vi "VP_NanoPositioner_FPGA.vi"() -> ()   [LabVIEW 2015]
uses:
  FPGA states.ctl
  FPGA Commands.ctl
  <vilib>/Platform/TimedLoop/XDataNode/timing_clust.ctl
  <vilib>/Platform/TimedLoop/XDataNode/nitl_modes.ctl
  <vilib>/Platform/TimedLoop/XDataNode/wakeup.ctl
  Control X Up Down Ramp.ctl
  Control Y Up Down Ramp.ctl
  Detector_Trigger_Control.ctl
  <vilib>/rvi/Emulation/niFpgaGetClockAttributes.vi
  <vilib>/rvi/Emulation/niFpgaSctlEmulationGetInTimedLoop.vi
  <vilib>/rvi/Emulation/niFpgaEmulationReportErrorSimple.vi
  <vilib>/rvi/eio/common/nirviEmuTemplateMethod_errors.vi
  <vilib>/rvi/Emulation/niFpgaProcessEmulError.vi
  <vilib>/rvi/Emulation/niFpgaCriticalErrorInLSC.vi
  <vilib>/rvi/interface/RandomDataEmulation/niFpgaRandomDataHandleErrors.vi
  <vilib>/eio/EIONode/EIONode.xnode
  <vilib>/rvi/DataTransferAndStorage/Container/XNode/niFpgaContainer.xnode
  <vilib>/rvi/interface/RandomDataEmulation/nirviRandomDataFpgaReadWriteTemplate.vi
  <vilib>/rvi/Analysis/measure/butterworth/XNode/niFpgaButterworthFilter.xnode
  <vilib>/Platform/TimedLoop/XDataNode/XDataNode.xnode
  <vilib>/Platform/TimedLoop/XDataNode/XDNodeRunTimeDep.lvlib
panel:
  out "Fly scan completed":bool
  out "Y scan done":bool=TRUE
  out "X scan done":bool=TRUE
  out "Wait error":errorcluster
  out "Shutdown error":errorcluster
  out "FPGA error monitor":errorcluster
  out "Run Loop error":errorcluster
  in  "Wait timer (ms)":u16=50 caption="Count(mSec)"
  in  "New FPGA command":bool
  in  "FPGA command":T1
  out "FPGA state":T2
  out "End Run Error":errorcluster
  out "Number of Data Strings 2":i32
  out "Measured Data Trigger Time Period (Ticks)":u32
  in  "Data Trigger Time Period (uSec)":u32 caption="Detector Trigger Time Period (uSec)"
  out "Trigger for Data":fxp<+/-,58,25>
  out "Fly Scan Running":bool
  in  "Fly Scan":bool
  out "If True End Y Down Ramp":bool
  in  "Y Ramp Drop Size (nm)":fxp<+/-,16,16>
  out "Ramp Mid Range":bool
  out "If True End Up Ramp":bool
  out "Start or middle":bool=TRUE
  in  "Y Start Marker (nm)":fxp<+/-,58,25> format="%#_55g"
  out "Y Ramp Slope":fxp<+,48,16>
  in  "Y Ramp End (nm)":fxp<+/-,16,16>
  in  "Y Ramp Start (nm)":fxp<+/-,16,16>
  in  "Y Ramp Period (usec)":fxp<+,32,32>
  in  "X Ramp Period (usec)":fxp<+,32,32>
  in  "X Ramp End (nm)":fxp<+/-,16,16>
  in  "X Ramp Start (nm)":fxp<+/-,16,16>
  out "If True End X Down Ramp":bool
  out "X Ramp Mid Range":bool
  out "If True End X Up Ramp":bool
  out "Y Ramp Drop":bool
  out "Next Do Down Ramp":bool
  out "Continue Run":bool
  in  "X Start Marker (nm)":fxp<+/-,58,25>
  out "X Ramp Slope":fxp<+,48,16> format="%.37g"
  in  "DT Reset":bool
  in  "DT Duty Cycle (periods)":fxp<+,32,0>=0.5 caption="DT duty cycle (periods)"
  in  "DT Reference DC Offset (V)":fxp<+/-,16,16>
  in  "DT Reference Amplitude (V)":fxp<+/-,40,17>
  in  "DT Phase Offset (periods)":fxp<+,32,0>
  in  "DT Frequency (periods/tick)":fxp<+,32,0>=0.0002500000409781933
  in  "Trigger Wave Generator":T3(ring)
  out "If True End Trigger Low":bool
  in  "Trigger Low Level (V)":fxp<+/-,20,5>=-5.0
  in  "Trigger High Level (V)":fxp<+/-,20,5>=5.0
  out "If True End Trigger High":bool
  out "Trigger Mid High":bool
  in  "Trigger Low Period (usec)":fxp<+/-,64,45>
  in  "Trigger High Period (usec)":fxp<+/-,64,45>
  out "Measured Z Reference Time Period (Ticks)":u32
  in  "Z Reference Time Period (uSec)":u32
  in  "Z White Noise Amplitude":u16=32767
  in  "Z White Noise Seed":u32=4
  in  "Z Phase Offset (periods)":fxp<+,32,0>
  in  "Z Frequency (periods/tick)":fxp<+,32,0>=0.0002500000409781933
  in  "Z Reference DC Offset (nm)":fxp<+/-,16,16>
  in  "Z Reference Amplitude (nm)":fxp<+/-,40,17>
  in  "Z Reference Reset":bool
  in  "Z Reference Wave Selection":T4(ring)
  in  "Y White Noise Amplitude":u16=32767
  in  "Y White Noise Seed":u32=4
  out "Measured Y Reference Time Period (Ticks)":u32
  in  "Y Reference Time Period (uSec)":u32
  in  "Y Reference Reset":bool
  in  "Y Reference Wave Selection":T5(ring)
  in  "Detector Trigger Lower Limit (V)":fxp<+/-,20,5>=-5.0
  out "Detector Trigger In Range?":bool
  in  "Detector Trigger Upper Limit (V)":fxp<+/-,20,5>=5.0
  out "Detector Trigger (V)":fxp<+/-,20,5> format="%.29g"
  out "Measured Detector Trigger Time Period (Ticks)":u32
  in  "Detector Trigger Time Period (uSec)":u32
  out "Measured Trigger Gen Time Period (Ticks)":u32
  in  "Trigger Generation Time Period (uSec)":u32
  in  "Reference Signal Source":T6(ring)
  in  "Z-Stage Scaling Direction":fxp<+/-,3,3>=-1.0
  in  "Y-Stage Scaling Direction":fxp<+/-,3,3>=-1.0
  in  "Y Phase Offset (periods)":fxp<+,32,0>
  in  "Y Frequency (periods/tick)":fxp<+,32,0>=0.0002500000409781933
  in  "Optics and or Sample Stage":T7(ring)
  out "Z Stage External Reference (nm)":fxp<+/-,58,25>
  in  "Mod 3 AI2 V to nm Scaling":fxp<+,47,18>
  out "Mod 8 Input AI2 (V)":fxp<+/-,24,5>
  out "Y Stage External Reference (nm)":fxp<+/-,58,25>
  in  "Mod 3 AI1 V to nm Scaling":fxp<+,47,18>
  out "Mod 8 Input AI1 (V)":fxp<+/-,24,5>
  in  "Sample Z Stage Resolution (nm)":fxp<+,33,3>=0.001000046730041504
  in  "Sample Y Stage Resolution (nm)":fxp<+,33,3>=0.001000046730041504
  in  "Sample X Stage Resolution (nm)":fxp<+,33,3>=0.001000046730041504
  out "Sample Z Stage Displacement (nm)":fxp<+/-,58,25>
  out "Sample Z Stage Displacement raw (nm)":fxp<+/-,64,35> format="%.62g"
  out "Sample Y Stage Displacement (nm)":fxp<+/-,58,25>
  out "Sample Y Stage Displacement raw (nm)":fxp<+/-,64,35> format="%.41g"
  out "Sample X Stage Displacement raw (nm)":fxp<+/-,64,35> format="%.62g"
  out "Sample X Stage Displacement (nm)":fxp<+/-,58,25>
  in  "Reset Sample Z":bool
  out "32 bit Count Sample  Z":i32
  in  "Reset Sample Y":bool
  out "32 bit Count Sample  Y":i32
  in  "Reset Sample X":bool
  out "32 bit Count Sample X":i32
  out "Mod6/DIO3":bool
  out "Mod6/DIO2":bool
  out "Mod5/DIO3":bool
  out "Mod5/DIO2":bool
  out "Mod4/DIO3":bool
  out "Mod4/DIO2":bool
  out "Measured Analog Input Time Period (Ticks)":u32
  in  "Analog Input Time Period (uSec)":u32
  out "X Stage External Reference (nm)":fxp<+/-,58,25>
  in  "Mod 3 AI0 V to nm Scaling":fxp<+,47,18>
  out "Mod 3 Input AI0 (V)":fxp<+/-,24,5>
  out "Kxz Output, Kxz*ex (V)":fxp<+/-,58,25> format="%.31g"
  out "Kyz Output, Kyz*ey (V)":fxp<+/-,58,25> format="%.31g"
  in  "b02(2) yz1":fxp<+/-,64,9>[](array[numeric])=[0.0, 0.0, 0.0, 0.0, 0.0, 0.0, 0.0, 0.0, 0.0, 0.0, 0.0, 0.0, 0.0, 0.0, 0.0, 0.0, 0.0, 0.0, 0.0, 0.0]
  in  "b01(2) yz1":fxp<+/-,64,9>[](array[numeric])=[0.0, 0.0, 0.0, 0.0, 0.0, 0.0, 0.0, 0.0, 0.0, 0.0, 0.0, 0.0, 0.0, 0.0, 0.0, 0.0, 0.0, 0.0, 0.0, 0.0]
  in  "-a02(2) yz1":fxp<+/-,64,9>[](array[numeric])=[0.0, 0.0, 0.0, 0.0, 0.0, 0.0, 0.0, 0.0, 0.0, 0.0, 0.0, 0.0, 0.0, 0.0, 0.0, 0.0, 0.0, 0.0, 0.0, 0.0]
  in  "-a01(2) yz1":fxp<+/-,64,9>[](array[numeric])=[0.0, 0.0, 0.0, 0.0, 0.0, 0.0, 0.0, 0.0, 0.0, 0.0, 0.0, 0.0, 0.0, 0.0, 0.0, 0.0, 0.0, 0.0, 0.0, 0.0]
  in  "sos gain SF Controller yz1":fxp<+/-,42,9>
  in  "b02(2) xz1":fxp<+/-,64,9>[](array[numeric])=[0.0, 0.0, 0.0, 0.0, 0.0, 0.0, 0.0, 0.0, 0.0, 0.0, 0.0, 0.0, 0.0, 0.0, 0.0, 0.0, 0.0, 0.0, 0.0, 0.0]
  in  "b01(2) xz1":fxp<+/-,64,9>[](array[numeric])=[0.0, 0.0, 0.0, 0.0, 0.0, 0.0, 0.0, 0.0, 0.0, 0.0, 0.0, 0.0, 0.0, 0.0, 0.0, 0.0, 0.0, 0.0, 0.0, 0.0]
  in  "-a02(2) xz1":fxp<+/-,64,9>[](array[numeric])=[0.0, 0.0, 0.0, 0.0, 0.0, 0.0, 0.0, 0.0, 0.0, 0.0, 0.0, 0.0, 0.0, 0.0, 0.0, 0.0, 0.0, 0.0, 0.0, 0.0]
  in  "-a01(2) xz1":fxp<+/-,64,9>[](array[numeric])=[0.0, 0.0, 0.0, 0.0, 0.0, 0.0, 0.0, 0.0, 0.0, 0.0, 0.0, 0.0, 0.0, 0.0, 0.0, 0.0, 0.0, 0.0, 0.0, 0.0]
  in  "sos gain SF Controller xz1":fxp<+/-,42,9>
  out "Kzy Output, Kzy*ez (V)":fxp<+/-,58,25> format="%.31g"
  out "Kxy Output, Kxy*ex (V)":fxp<+/-,58,25> format="%.31g"
  in  "b02(2) zy1":fxp<+/-,64,9>[](array[numeric])=[0.0, 0.0, 0.0, 0.0, 0.0, 0.0, 0.0, 0.0, 0.0, 0.0, 0.0, 0.0, 0.0, 0.0, 0.0, 0.0, 0.0, 0.0, 0.0, 0.0]
  in  "b01(2) zy1":fxp<+/-,64,9>[](array[numeric])=[0.0, 0.0, 0.0, 0.0, 0.0, 0.0, 0.0, 0.0, 0.0, 0.0, 0.0, 0.0, 0.0, 0.0, 0.0, 0.0, 0.0, 0.0, 0.0, 0.0]
  in  "-a02(2) zy1":fxp<+/-,64,9>[](array[numeric])=[0.0, 0.0, 0.0, 0.0, 0.0, 0.0, 0.0, 0.0, 0.0, 0.0, 0.0, 0.0, 0.0, 0.0, 0.0, 0.0, 0.0, 0.0, 0.0, 0.0]
  in  "-a01(2) zy1":fxp<+/-,64,9>[](array[numeric])=[0.0, 0.0, 0.0, 0.0, 0.0, 0.0, 0.0, 0.0, 0.0, 0.0, 0.0, 0.0, 0.0, 0.0, 0.0, 0.0, 0.0, 0.0, 0.0, 0.0]
  in  "sos gain SF Controller zy1":fxp<+/-,42,9>
  in  "b02(2) xy1":fxp<+/-,64,9>[](array[numeric])=[0.0, 0.0, 0.0, 0.0, 0.0, 0.0, 0.0, 0.0, 0.0, 0.0, 0.0, 0.0, 0.0, 0.0, 0.0, 0.0, 0.0, 0.0, 0.0, 0.0]
  in  "b01(2) xy1":fxp<+/-,64,9>[](array[numeric])=[0.0, 0.0, 0.0, 0.0, 0.0, 0.0, 0.0, 0.0, 0.0, 0.0, 0.0, 0.0, 0.0, 0.0, 0.0, 0.0, 0.0, 0.0, 0.0, 0.0]
  in  "-a02(2) xy1":fxp<+/-,64,9>[](array[numeric])=[0.0, 0.0, 0.0, 0.0, 0.0, 0.0, 0.0, 0.0, 0.0, 0.0, 0.0, 0.0, 0.0, 0.0, 0.0, 0.0, 0.0, 0.0, 0.0, 0.0]
  in  "-a01(2) xy1":fxp<+/-,64,9>[](array[numeric])=[0.0, 0.0, 0.0, 0.0, 0.0, 0.0, 0.0, 0.0, 0.0, 0.0, 0.0, 0.0, 0.0, 0.0, 0.0, 0.0, 0.0, 0.0, 0.0, 0.0]
  in  "sos gain SF Controller xy1":fxp<+/-,42,9>
  out "Kzx Output, Kzx*ez (V)":fxp<+/-,58,25> format="%.31g"
  in  "b02(2) zx1":fxp<+/-,64,9>[](array[numeric])=[0.0, 0.0, 0.0, 0.0, 0.0, 0.0, 0.0, 0.0, 0.0, 0.0, 0.0, 0.0, 0.0, 0.0, 0.0, 0.0, 0.0, 0.0, 0.0, 0.0]
  in  "b01(2) zx1":fxp<+/-,64,9>[](array[numeric])=[0.0, 0.0, 0.0, 0.0, 0.0, 0.0, 0.0, 0.0, 0.0, 0.0, 0.0, 0.0, 0.0, 0.0, 0.0, 0.0, 0.0, 0.0, 0.0, 0.0]
  in  "-a02(2) zx1":fxp<+/-,64,9>[](array[numeric])=[0.0, 0.0, 0.0, 0.0, 0.0, 0.0, 0.0, 0.0, 0.0, 0.0, 0.0, 0.0, 0.0, 0.0, 0.0, 0.0, 0.0, 0.0, 0.0, 0.0]
  in  "-a01(2) zx1":fxp<+/-,64,9>[](array[numeric])=[0.0, 0.0, 0.0, 0.0, 0.0, 0.0, 0.0, 0.0, 0.0, 0.0, 0.0, 0.0, 0.0, 0.0, 0.0, 0.0, 0.0, 0.0, 0.0, 0.0]
  in  "sos gain SF Controller zx1":fxp<+/-,42,9>
  out "Kyx Output, Kyx*ey (V)":fxp<+/-,58,25> format="%.31g"
  in  "b02(2) yx1":fxp<+/-,64,9>[](array[numeric])=[0.0, 0.0, 0.0, 0.0, 0.0, 0.0, 0.0, 0.0, 0.0, 0.0, 0.0, 0.0, 0.0, 0.0, 0.0, 0.0, 0.0, 0.0, 0.0, 0.0]
  in  "b01(2) yx1":fxp<+/-,64,9>[](array[numeric])=[0.0, 0.0, 0.0, 0.0, 0.0, 0.0, 0.0, 0.0, 0.0, 0.0, 0.0, 0.0, 0.0, 0.0, 0.0, 0.0, 0.0, 0.0, 0.0, 0.0]
  in  "-a02(2) yx1":fxp<+/-,64,9>[](array[numeric])=[0.0, 0.0, 0.0, 0.0, 0.0, 0.0, 0.0, 0.0, 0.0, 0.0, 0.0, 0.0, 0.0, 0.0, 0.0, 0.0, 0.0, 0.0, 0.0, 0.0]
  in  "-a01(2) yx1":fxp<+/-,64,9>[](array[numeric])=[0.0, 0.0, 0.0, 0.0, 0.0, 0.0, 0.0, 0.0, 0.0, 0.0, 0.0, 0.0, 0.0, 0.0, 0.0, 0.0, 0.0, 0.0, 0.0, 0.0]
  in  "sos gain SF Controller yx1":fxp<+/-,42,9>
  in  "X-Stage Scaling Direction":fxp<+/-,3,3>=-1.0
  in  "Z-Stage nm to V Scaling":fxp<+/-,32,12>
  in  "Y-Stage nm to V Scaling":fxp<+/-,32,12>
  in  "X-Stage nm to V Scaling":fxp<+/-,32,12>
  out "Kxx Output, Kxx*ex (V)":fxp<+/-,58,25>
  out "Kyy Output, Kyy*ey (V)":fxp<+/-,58,25>
  out "Kzz Output, Kzz*ez (V)":fxp<+/-,58,25>
  in  "sos gain SF Controller xx1":fxp<+/-,42,9>
  in  "-a01(2) xx1":fxp<+/-,64,9>[](array[numeric])=[0.0, 0.0, 0.0, 0.0, 0.0, 0.0, 0.0, 0.0, 0.0, 0.0, 0.0, 0.0, 0.0, 0.0, 0.0, 0.0, 0.0, 0.0, 0.0, 0.0]
  in  "-a02(2) xx1":fxp<+/-,64,9>[](array[numeric])=[0.0, 0.0, 0.0, 0.0, 0.0, 0.0, 0.0, 0.0, 0.0, 0.0, 0.0, 0.0, 0.0, 0.0, 0.0, 0.0, 0.0, 0.0, 0.0, 0.0]
  in  "b01(2) xx1":fxp<+/-,64,9>[](array[numeric])=[0.0, 0.0, 0.0, 0.0, 0.0, 0.0, 0.0, 0.0, 0.0, 0.0, 0.0, 0.0, 0.0, 0.0, 0.0, 0.0, 0.0, 0.0, 0.0, 0.0]
  in  "b02(2) xx1":fxp<+/-,64,9>[](array[numeric])=[0.0, 0.0, 0.0, 0.0, 0.0, 0.0, 0.0, 0.0, 0.0, 0.0, 0.0, 0.0, 0.0, 0.0, 0.0, 0.0, 0.0, 0.0, 0.0, 0.0]
  in  "sos gain SF Controller yy1":fxp<+/-,42,9>
  in  "-a01(2) yy1":fxp<+/-,64,9>[](array[numeric])=[0.0, 0.0, 0.0, 0.0, 0.0, 0.0, 0.0, 0.0, 0.0, 0.0, 0.0, 0.0, 0.0, 0.0, 0.0, 0.0, 0.0, 0.0, 0.0, 0.0]
  in  "-a02(2) yy1":fxp<+/-,64,9>[](array[numeric])=[0.0, 0.0, 0.0, 0.0, 0.0, 0.0, 0.0, 0.0, 0.0, 0.0, 0.0, 0.0, 0.0, 0.0, 0.0, 0.0, 0.0, 0.0, 0.0, 0.0]
  in  "b01(2) yy1":fxp<+/-,64,9>[](array[numeric])=[0.0, 0.0, 0.0, 0.0, 0.0, 0.0, 0.0, 0.0, 0.0, 0.0, 0.0, 0.0, 0.0, 0.0, 0.0, 0.0, 0.0, 0.0, 0.0, 0.0]
  in  "b02(2) yy1":fxp<+/-,64,9>[](array[numeric])=[0.0, 0.0, 0.0, 0.0, 0.0, 0.0, 0.0, 0.0, 0.0, 0.0, 0.0, 0.0, 0.0, 0.0, 0.0, 0.0, 0.0, 0.0, 0.0, 0.0]
  in  "sos gain SF Controller zz1":fxp<+/-,42,9>
  in  "-a01(2) zz1":fxp<+/-,64,9>[](array[numeric])=[0.0, 0.0, 0.0, 0.0, 0.0, 0.0, 0.0, 0.0, 0.0, 0.0, 0.0, 0.0, 0.0, 0.0, 0.0, 0.0, 0.0, 0.0, 0.0, 0.0]
  in  "-a02(2) zz1":fxp<+/-,64,9>[](array[numeric])=[0.0, 0.0, 0.0, 0.0, 0.0, 0.0, 0.0, 0.0, 0.0, 0.0, 0.0, 0.0, 0.0, 0.0, 0.0, 0.0, 0.0, 0.0, 0.0, 0.0]
  in  "b01(2) zz1":fxp<+/-,64,9>[](array[numeric])=[0.0, 0.0, 0.0, 0.0, 0.0, 0.0, 0.0, 0.0, 0.0, 0.0, 0.0, 0.0, 0.0, 0.0, 0.0, 0.0, 0.0, 0.0, 0.0, 0.0]
  in  "b02(2) zz1":fxp<+/-,64,9>[](array[numeric])=[0.0, 0.0, 0.0, 0.0, 0.0, 0.0, 0.0, 0.0, 0.0, 0.0, 0.0, 0.0, 0.0, 0.0, 0.0, 0.0, 0.0, 0.0, 0.0, 0.0]
  in  "Scaling mV to V":fxp<+,33,10>=0.0009765625
  in  "System Loop Type":enum16{"Open Loop", "Closed Loop"}(ring)
  in  "Timeout FPGA FIFO1":i32=40000000
  out "FIFO Timed Out":bool
  out "Number of Data Strings":i32
  in  "Y Reference DC Offset (nm)":fxp<+/-,16,16>
  in  "X Reference DC Offset (nm)":fxp<+/-,16,16>
  in  "Y Reference Amplitude (nm)":fxp<+/-,40,17>
  out "Z Stage Reference (nm)":fxp<+/-,58,25> format="%.41g"
  out "Y Stage Reference (nm)":fxp<+/-,58,25> format="%.41g"
  out "Optics Z Stage Displacement (nm)":fxp<+/-,58,25>
  out "Optics Z Stage Displacement raw (nm)":fxp<+/-,64,35>
  in  "Optics Z Stage Resolution (nm)":fxp<+,33,3>=0.001000046730041504
  in  "Reset Optics Z":bool
  out "32 bit Count Optics  Z":i32
  out "Mod6/DIO1":bool
  out "Mod6/DIO0":bool
  out "Optics Y Stage Displacement (nm)":fxp<+/-,58,25>
  out "Optics Y Stage Displacement raw (nm)":fxp<+/-,64,35>
  in  "Optics Y Stage Resolution (nm)":fxp<+,33,3>=0.001000046730041504
  in  "Reset Optics Y":bool
  out "32 bit Count Optics  Y":i32
  out "Mod5/DIO1":bool
  out "Mod5/DIO0":bool
  out "Z-Stage Input In Range?":bool
  out "Y-Stage Input In Range?":bool
  in  "Controller Output Lower Limit":fxp<+/-,20,5>=-5.0
  out "X-Stage Input In Range?":bool
  in  "Controller Output Upper Limit":fxp<+/-,20,5>=5.0
  in  "X White Noise Amplitude":u16=32767
  in  "X White Noise Seed":u32=4
  in  "X Reference Reset":bool
  in  "X Reference Wave Selection":T8(ring)
  out "Measured Counter Time Period (Ticks)":u32
  out "Measured Datalog Time Period (Ticks)":u32
  out "Measured Plant Output Time Period (Ticks)":u32
  out "Measured Controller Output Time Period (Ticks)":u32
  out "Measured Controller Time Period (Ticks)":u32
  out "Measured X Reference Time Period (Ticks)":u32
  out "Optics X Stage Displacement raw (nm)":fxp<+/-,64,35>
  in  "Optics X Stage Resolution (nm)":fxp<+,33,3>=0.001000046730041504 format="%#_31g"
  in  "Plant Output Time Period (uSec)":u32
  out "Optics X Stage Displacement (nm)":fxp<+/-,58,25>
  in  "Reset Optics X":bool
  out "32 bit Count Optics X":i32
  out "Mod4/DIO1":bool
  out "Mod4/DIO0":bool
  out "Start Run Error":errorcluster
  out "stop case":bool
  in  "Controller Output Time Period (uSec)":u32
  in  "Datalog Cases":T9(ring)
  out "PI Z-Stage Input (V)":fxp<+/-,20,5> format="%.29g"
  out "PI Y-Stage Input (V)":fxp<+/-,20,5> format="%.29g"
  out "PI X-Stage Input (V)":fxp<+/-,20,5> format="%.29g"
  in  "Controller Time Period (uSec)":u32
  in  "Datalog Time Period (uSec)":u32
  in  "X Reference Time Period (uSec)":u32
  in  "X Reference Amplitude (nm)":fxp<+/-,40,17>
  out "X Stage Reference (nm)":fxp<+/-,58,25> format="%.41g"
  out "FIFO Timed Out?":bool
  in  "X Phase Offset (periods)":fxp<+,32,0>
  in  "X Frequency (periods/tick)":fxp<+,32,0>=0.0002500000409781933
types:
  T1 = typedef "FPGA Commands.ctl" = enum16{"Start Scan", "Shutdown"}
  T2 = typedef "FPGA states.ctl" = enum16{"Wait", "Start Run", "Run", "End Run", "Shutdown"}
  T3 = enum16{"Custom Square Wave ", "Square Wave 1", "Square Wave 2"}
  T4 = enum16{"Constant", "Sine Wave", "Sawtooth Wave", "Square Wave", "Filtered White Noise"}
  T5 = enum16{"Constant", "Sine Wave", "Custom Ramp Wave", "Filtered White Noise"}
  T6 = enum16{"FPGA Generated Reference", "External Reference"}
  T7 = enum16{"Optics Stage Only", "Optics and Sample Stage"}
  T8 = enum16{"Constant", "Sine Wave", "Custom Up Down Ramp", "Filtered White Noise"}
  T9 = enum16{"Data Log 1", "Data Log 2", "Data Log 3", "Data Log 4", "Data Log 5", "Data Log 6", "Data Log 7", "Data Log 8", "Data Log 9", "Data Log 10", "Data Log 11", "Data Log 12", "Data Log 13", "Data Log 14", "Data Log 15", "Data Log 16"}
  T10 = typedef "Control Y Up Down Ramp.ctl" = enum16{"Y Up Ramp", "Y Down Ramp"}
  T11 = typedef "Detector_Trigger_Control.ctl" = enum16{"Trigger High", "Trigger Low"}
  T12 = typedef "XDNodeRunTimeDep.lvlib/timing_clust.ctl" = cluster{"Expected End [f-1]":u64, "Actual End [f-1]":u64, "Finished Late? [f-1]":bool, "Expected End [i-1]":u64, "Actual End [i-1]":u64, "Finished Late? [i-1]":bool, "Expected Start [i]":u64, "Actual Start [i]":u64, "Expected Start [f]":u64, "Actual Start [f]":u64, "Source Name":string, "Structure Name":string, "Period":i64, "Deadline":i64, "Offset":i64, "Start":i64, "Priority":i32, "Timeout":i32, "Mode":T13, "Wakeup Reason":T14, "Error":errorcluster, "Source Type":string, "Secondary Source Type":string, "Global End Time":u64, "Global Start Time":u64, "Frame Duration":u64, "Iteration Duration":u64, "Assigned CPU":i32, "I/O Scan Engine Mode":u32}
  T13 = typedef "XDNodeRunTimeDep.lvlib/nitl_modes.ctl" = enum32{"No Change", "Process missed periods, maintain original phase", "Discard missed periods, maintain original phase", "Process missed periods, ignore original phase", "Discard missed periods, ignore original phase"}
  T14 = typedef "XDNodeRunTimeDep.lvlib/wakeup.ctl" = enum32{"Normal", "Aborted", "Asynchronous wakeup", "Timing source error", "Timed loop error", "Timeout"}
  T15 = typedef "Control X Up Down Ramp.ctl" = enum16{"X Up Ramp", "X Down Ramp"}
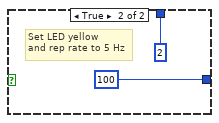
[diagram p2: hidden frame]
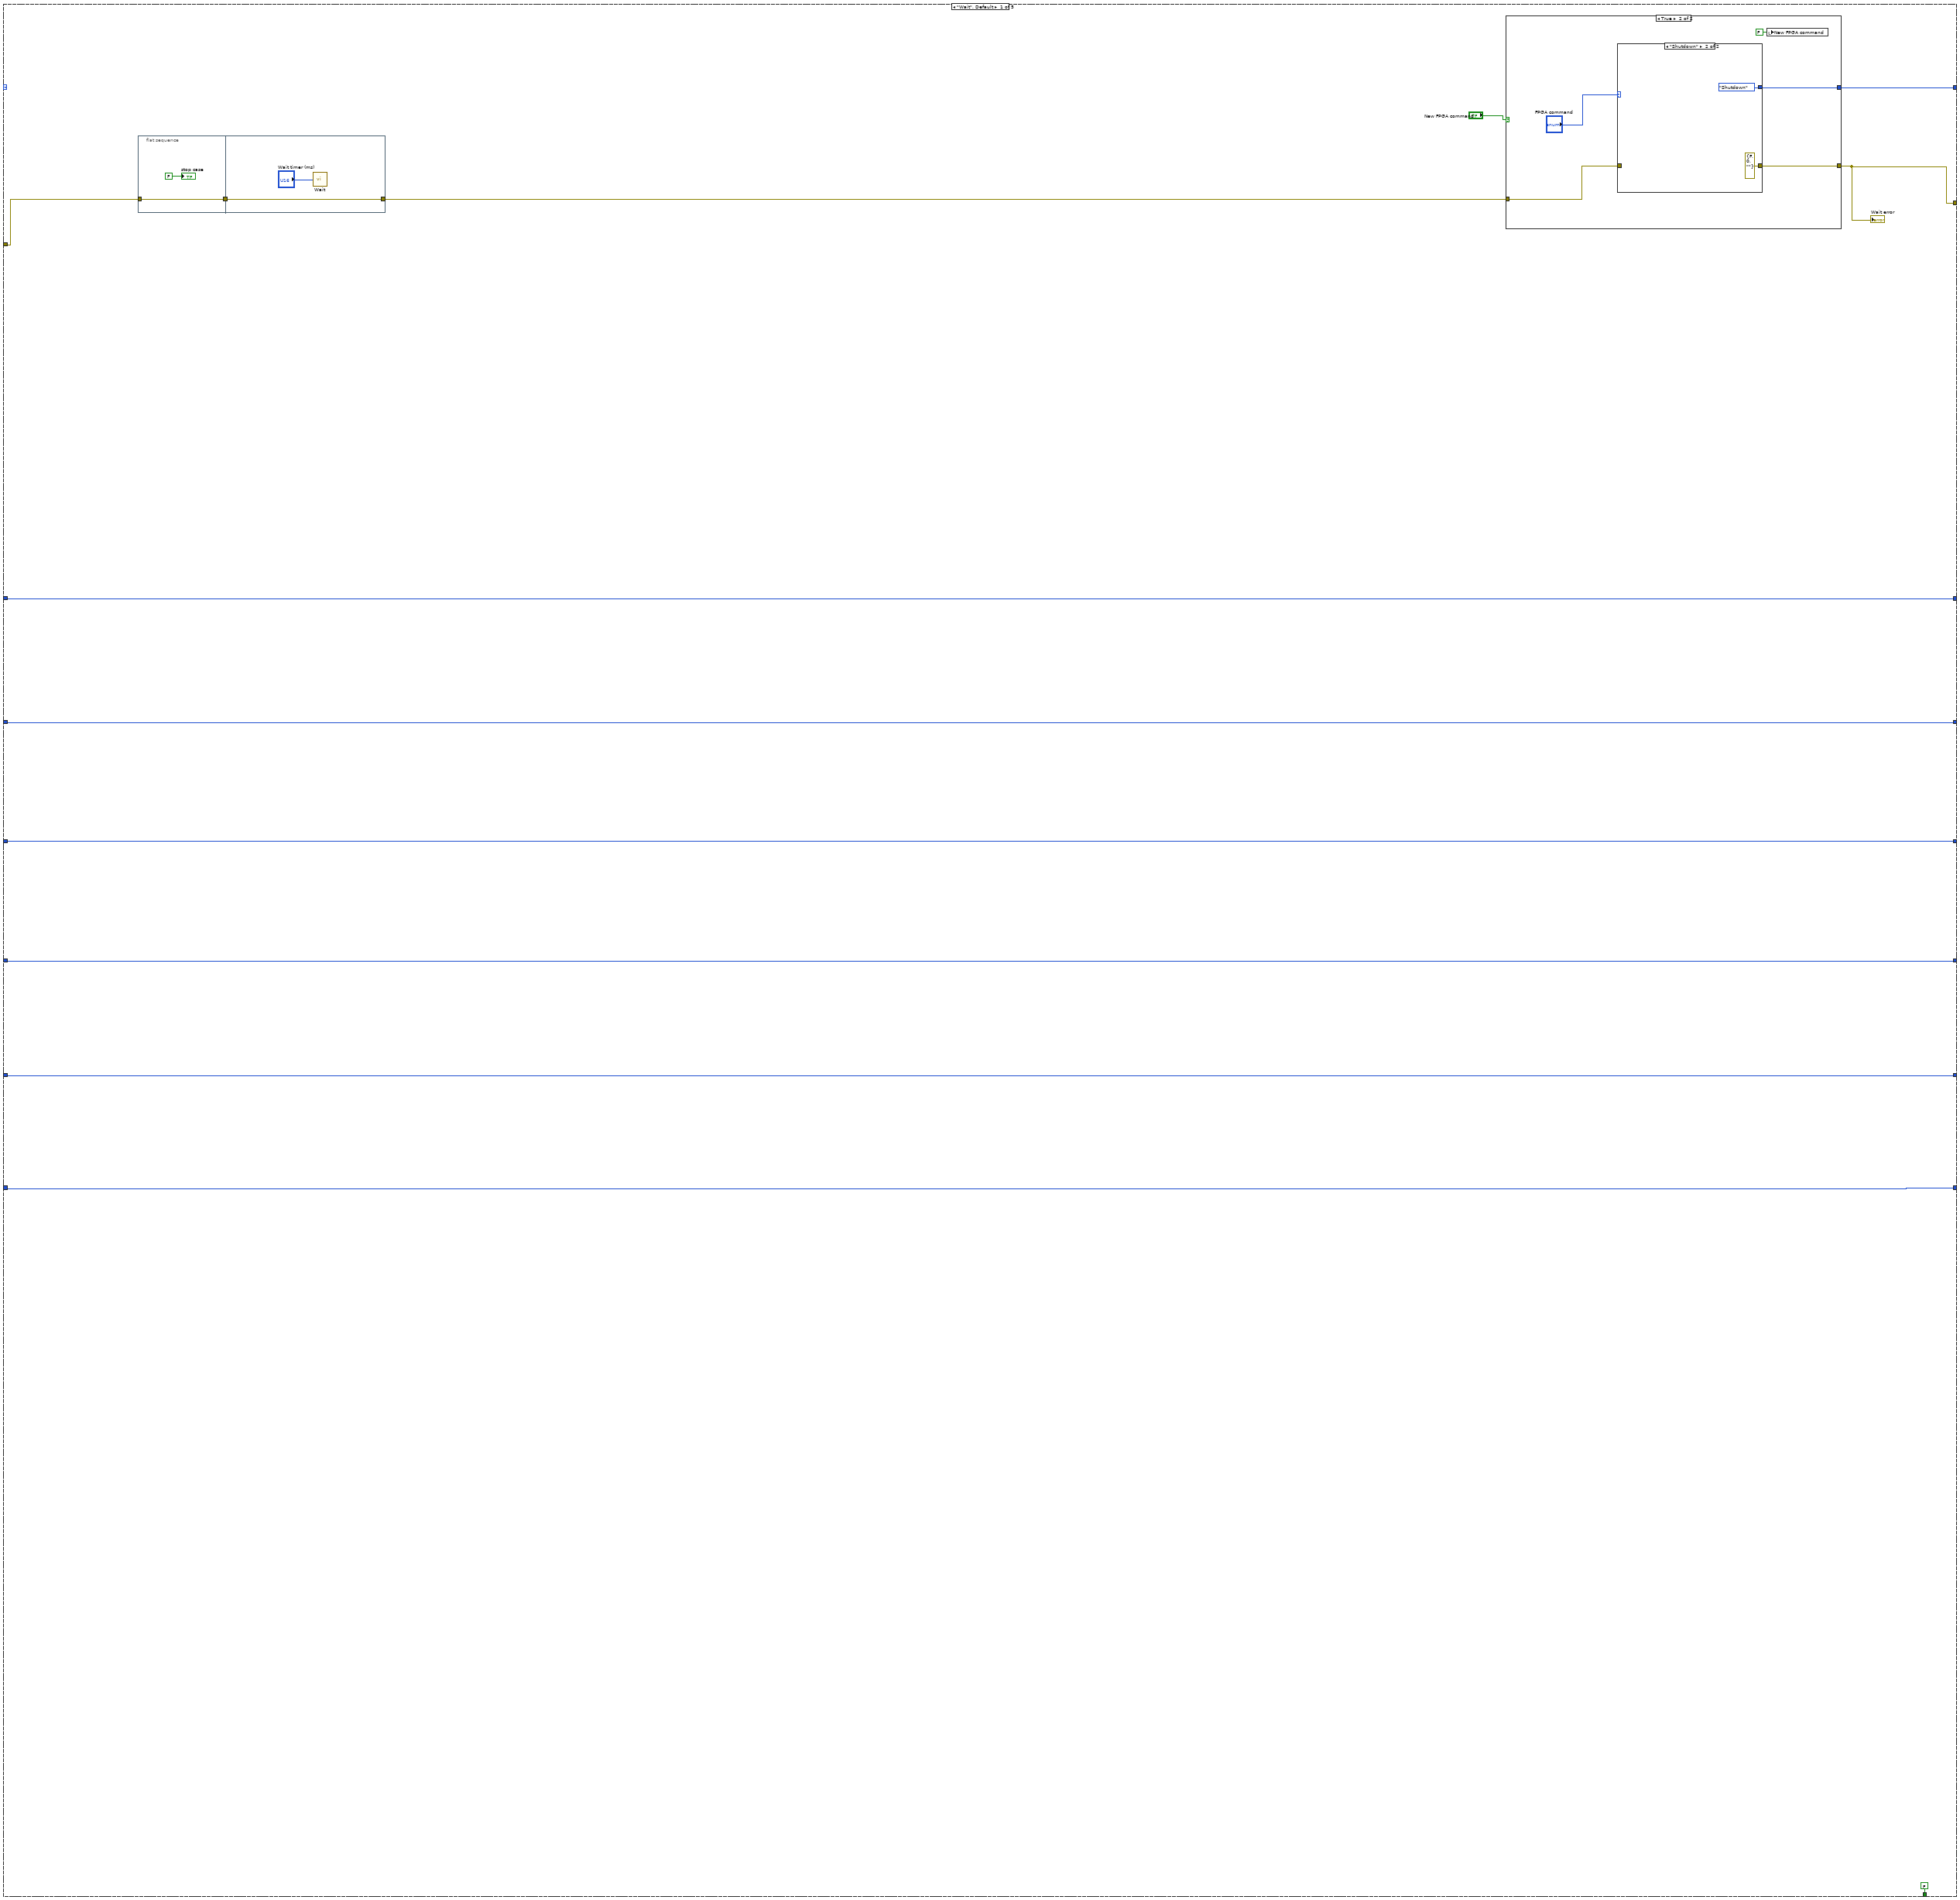
[diagram p3: hidden frame]
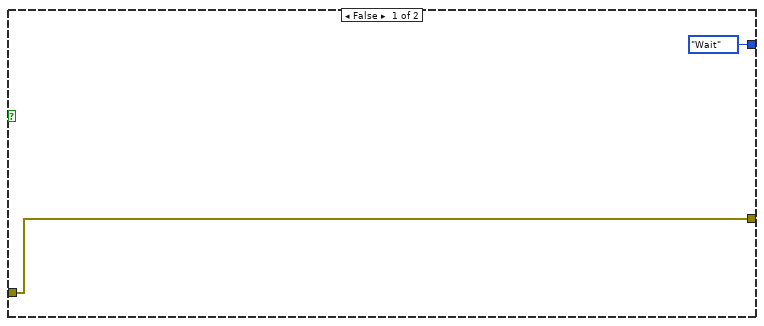
[diagram p4: hidden frame]
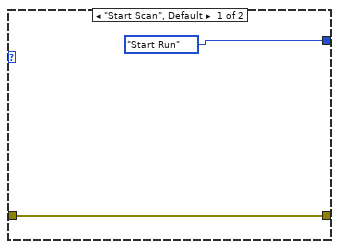
[diagram p5: hidden frame]
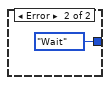
[diagram p6: hidden frame]
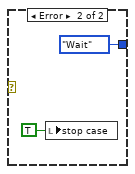
[diagram p8: hidden frame]
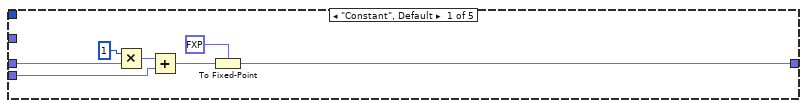
[diagram p9: hidden frame]
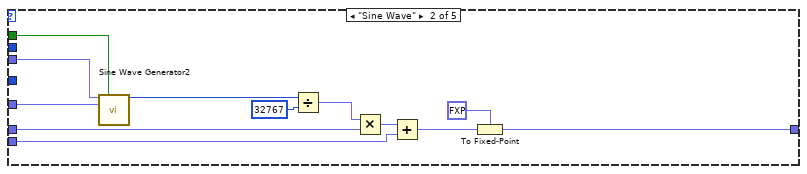
[diagram p10: hidden frame]
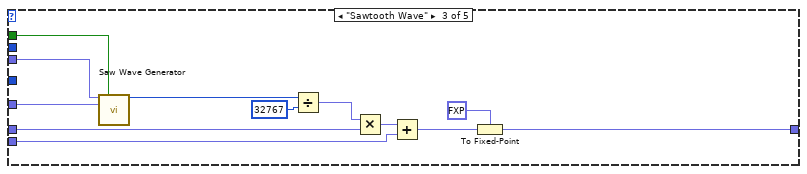
[diagram p11: hidden frame]
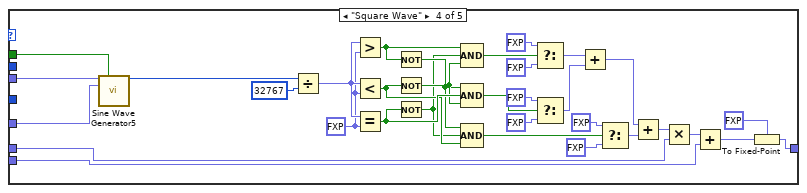
[diagram p12: hidden frame]
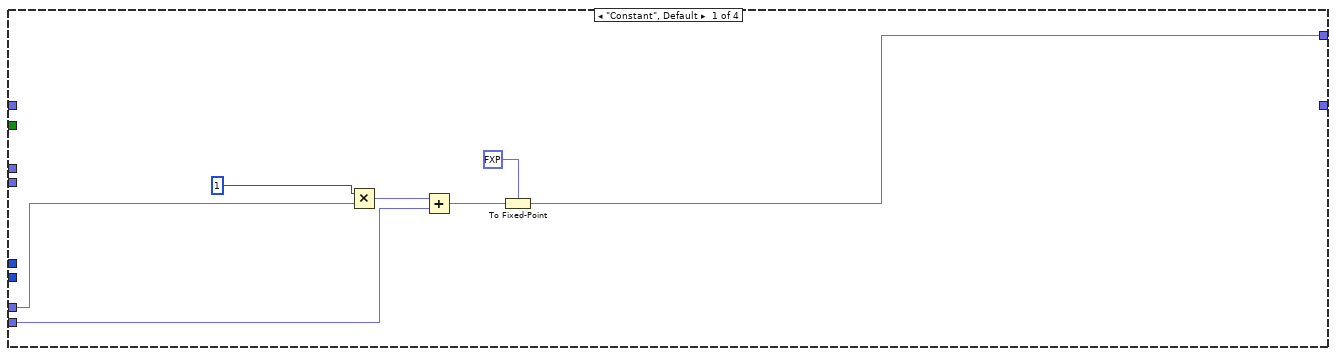
[diagram p13: hidden frame]
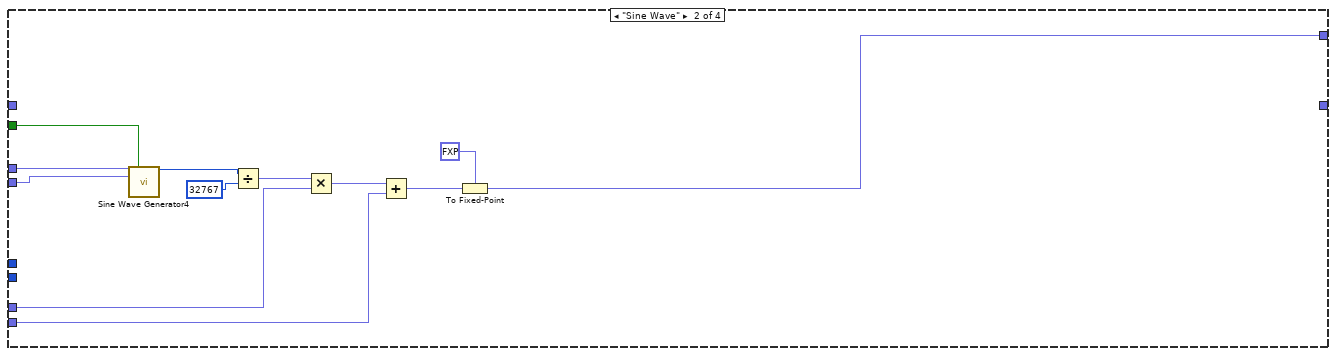
[diagram p14: hidden frame]
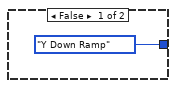
[diagram p15: hidden frame]
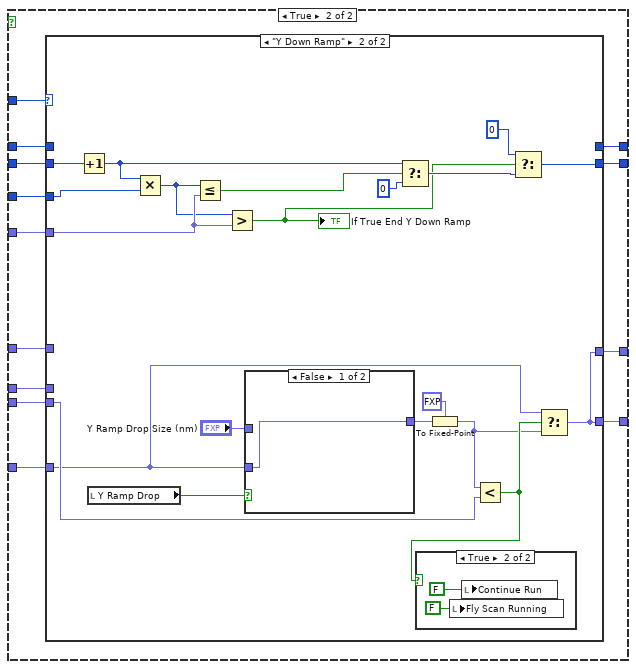
[diagram p16: hidden frame]
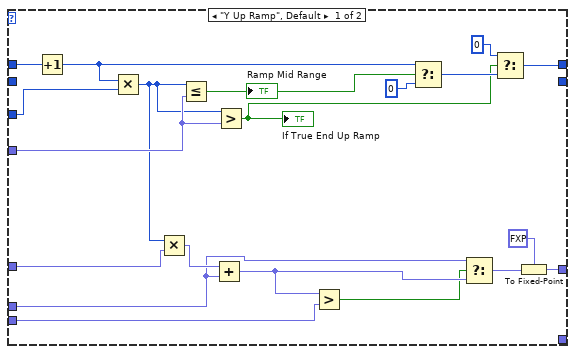
[diagram p17: hidden frame]
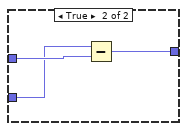
[diagram p18: hidden frame]
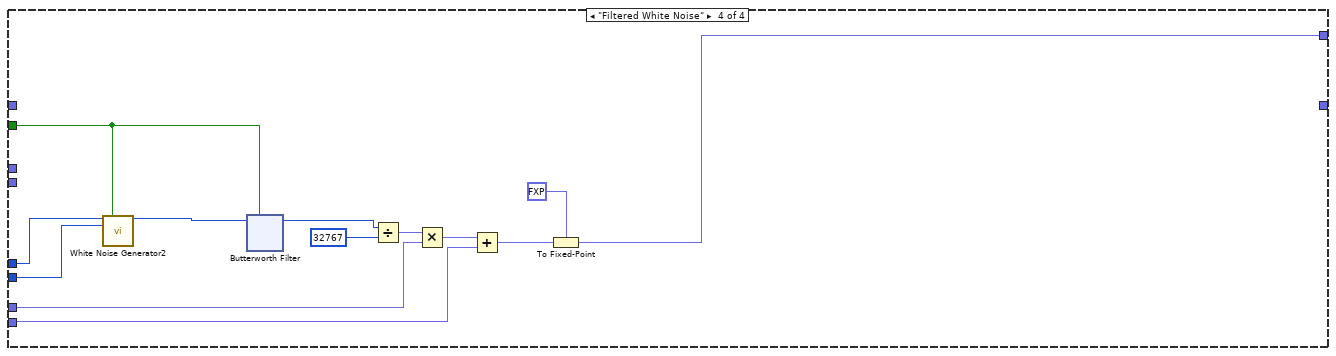
[diagram p20: hidden frame]
diagram:
  w5 = 0
  n1 = xnode "FPGA I/O Node"("error in"=errorcluster {"status"=FALSE, "code"=0, "source"=""} ("error IO"), "Mod3/Start"=TRUE ("I/O Item")) -> ("error out"=w2:errorcluster)  [unwired: 1 in, 1 out]
  n2 = while {
    tunnel: w2 -> [w19]
    shift-right: [w17] -> _
    shift-left: _ -> [w16]
    shift-right: [w14] -> _
    shift-left: u8 0 ("USER FPGA LED") -> [w12]
    stop <- FALSE stop-if-true
    # "Heartbeat Loop - monitors errors and relays status to RT and LED on cRIO"
    n3 = local read "Shutdown error"() -> (w21:errorcluster)
    n4 = local read "Run Loop error"() -> (w24:errorcluster)
    n5 = local read "Start Run Error"() -> (w23:errorcluster)
    n6 = local read "End Run Error"() -> (w20:errorcluster)
    n7 = local read "Wait error"() -> (w22:errorcluster)
    n8 = Merge Errors(w16, w24, w23, w22, w21, w20, w19) -> (w18:errorcluster)
    "FPGA error monitor" <- w18
    n9 = Unbundle By Name(w18) -> ("status"=w7:bool)
    n10 = Not Equal?(x=w12, y=u8 0) -> (x != y?=w10:bool)
    n11 = case shown="False" w7 {
      tunnel: [u16 500 ("Count(mSec)") u16 100 ("Count(mSec)")] -> w15
      tunnel: [u8 1 ("USER FPGA LED") u8 2 ("USER FPGA LED")] -> w8
      frame False {
        # "Set LED green \nand rep rate to 1 Hz"
      }
      frame True {
        # "Set LED yellow \nand rep rate to 5 Hz"
      }
    }
    n12 = Select(t=u8 0, s=w10, f=w8) -> (s? t:f=w14:u8)
    n13 = xnode "FPGA I/O Node"("USER FPGA LED"=w14) -> ("error out"=w17:errorcluster)  [unwired: 2 in, 1 out]
    n14 = call "Loop Timer12"("Count(mSec)"=w15) -> ()  [unwired: 1 out]
  }
  n15 = while {
    shift-right: [w43] -> _
    shift-left: FPGA_states."Wait" -> [w45]
    shift-right: [w42] -> _
    shift-left: w2 -> [w41]
    shift-right: [w29] -> _
    shift-left: w5 -> [w35]
    shift-right: [w30] -> _
    shift-left: w5 -> [w36]
    shift-right: [w31] -> _
    shift-left: w5 -> [w37]
    shift-right: [w34] -> _
    shift-left: w5 -> [w40]
    shift-right: [w33] -> _
    shift-left: w5 -> [w39]
    shift-right: [w32] -> _
    shift-left: w5 -> [w38]
    stop <- w44 stop-if-true
    n16 = case shown="\"Start Run\"" w45 {
      tunnel: [w56 w82 w99 w2049 w2059] -> w42
      tunnel: [FALSE FALSE FALSE FALSE TRUE] -> w44
      tunnel: [w58 w81 w100 FPGA_states."Wait" FPGA_states."Shutdown"] -> w43
      tunnel: w41 -> [w47 _ _ _ w2060]
      tunnel: w40 -> [w50 w74 w98 w2047 w2052]
      tunnel: w39 -> [w51 w75 w97 w2046 w2053]
      tunnel: w38 -> [w52 w76 w96 w2045 w2054]
      tunnel: w37 -> [w53 w77 w95 w2044 w2055]
      tunnel: w36 -> [w54 w78 w94 w2043 w2056]
      tunnel: w35 -> [w49 w79 w93 w2042 w2057]
      tunnel: [w50 w74 w92 w2047 w2052] -> w34
      tunnel: [w51 w75 w91 w2046 w2053] -> w33
      tunnel: [w52 w76 w90 w2045 w2054] -> w32
      tunnel: [w53 w77 w89 w2044 w2055] -> w31
      tunnel: [w54 w78 w88 w2043 w2056] -> w30
      tunnel: [w49 w79 w87 w2042 w2057] -> w29
      frame "Wait", Default {
        n17 = flat-sequence {
          tunnel: w47 -> [w59]
          tunnel: [w59] -> w48
          tunnel: [w61] -> w46
          tunnel: w48 -> [w61]
          frame #0 {
            "stop case" <- FALSE ("stop case")
          }
          frame #1 {
            n18 = call "Wait"("Count(mSec)"="Wait timer (ms)") -> ()  [unwired: 1 out]
          }
        }
        n19 = case shown="True" "New FPGA command" {
          tunnel: [FPGA_states."Wait" w69] -> w58
          tunnel: w46 -> [w64 w68]
          tunnel: [w64 w67] -> w56
          frame False {
          }
          frame True {
            n20 = case shown="\"Shutdown\"" "FPGA command" {
              tunnel: [FPGA_states."Start Run" FPGA_states."Shutdown"] -> w69
              tunnel: w68 -> [w70 _]
              tunnel: [w70 errorcluster {"status"=FALSE, "code"=0, "source"=""} ("error IO")] -> w67
              frame "Start Scan", Default {
              }
              frame "Shutdown" {
              }
            }
            n21 = local write "New FPGA command"(FALSE ("New FPGA command")) -> ()
          }
        }
        "Wait error" <- w56
      }
      frame "Start Run" {
        n22 = xnode "FPGA I/O Node"("Mod3/Start"=TRUE ("I/O Item")) -> ("error out"=w82:errorcluster)  [unwired: 2 in, 1 out]
        "Start Run Error" <- w82
        n23 = case shown="No Error" w82 {
          tunnel: [FPGA_states."Run" FPGA_states."Wait"] -> w81
          frame No Error {
            w84 = TRUE
            n24 = local write "X scan done"(w84) -> ()
            n25 = local write "Y scan done"(w84) -> ()
          }
          frame Error {
          }
        }
      }
      frame "Run" {
        w111 = errorcluster {"status"=FALSE, "code"=0, "source"=""}  # Error
        n26 = while {
          shift-right: [w1904] -> _
          shift-left: u32 0 ("f") -> [w1902]
          shift-right: [w1903] -> _
          shift-left: u32 0 -> [w1901]
          stop <- w1913 stop-if-true
          n27 = case shown="\"Custom Up Down Ramp\"" "X Reference Wave Selection" {
            tunnel: "X Frequency (periods/tick)" -> [_ w1935 _ _]
            tunnel: "X Phase Offset (periods)" -> [_ w1934 _ _]
            tunnel: "X Reference Reset" -> [_ w1932 _ w2031]
            tunnel: "X White Noise Seed" -> [_ _ _ w2033]
            tunnel: "X White Noise Amplitude" -> [_ _ _ w2030]
            tunnel: "X Reference Amplitude (nm)" -> [w1920 w1927 _ w2021]
            tunnel: "X Reference DC Offset (nm)" -> [w1919 w1926 _ w2022]
            tunnel: [w1918 w1925 w1939 w2024] -> w1906
            tunnel: [_ _ w1952 _] -> w1904
            tunnel: [_ _ w1951 _] -> w1903
            tunnel: w1902 -> [_ _ w1950 _]
            tunnel: w1901 -> [_ _ w1949 _]
            tunnel: "X Ramp Period (usec)" -> [_ _ w1948 _]
            tunnel: "X Ramp Start (nm)" -> [_ _ w1937 _]
            tunnel: "X Ramp End (nm)" -> [_ _ w1938 _]
            frame "Constant", Default {
              n28 = Multiply(x=i16 1 ("y"), y=w1920) -> (x*y=w1923:fxp<+/-,56,33>)
              n29 = Add(x=w1923, y=w1919) -> (x+y=w1922:fxp<+/-,56,33>)
              n30 = To Fixed-Point(fixed-point type=fxp<+/-,58,25> 0.0, number=w1922) -> (fixed-point=w1918:fxp<+/-,58,25>)
            }
            frame "Sine Wave" {
              n31 = call "Sine Wave Generator"("frequency (periods/tick)"=w1935, "reset"=w1932, "phase offset (periods)"=w1934) -> ("sine out"=w1933:i16)  [unwired: 12 in]
              n32 = Divide(x=w1933, y=i16 32767) -> (x/y=w1928:fxp<+/-,41,18>)
              n33 = Multiply(x=w1928, y=w1927) -> (x*y=w1930:fxp<+/-,64,35>)
              n34 = Add(x=w1930, y=w1926) -> (x+y=w1929:fxp<+/-,64,36>)
              n35 = To Fixed-Point(fixed-point type=fxp<+/-,58,25> 0.0, number=w1929) -> (fixed-point=w1925:fxp<+/-,58,25>)
            }
            frame "Custom Up Down Ramp" {
              n36 = local read "Next Do Down Ramp"() -> (w1944:bool)
              n37 = Subtract(x=w1937, y=w1938) -> (x-y=w1954:fxp<+/-,17,17>)
              n38 = Less?(x=w1937, y=w1938) -> (x < y?=w1943:bool)
              n39 = Absolute Value(x=w1954) -> (abs(x)=w1953:fxp<+,16,16>)
              n40 = Not(x=w1944) -> (.not. x?=w1945:bool)
              n41 = Divide(x=w1953, y=w1948) -> (x/y=w1955:fxp<+,48,16>)
              "X Ramp Slope" <- w1955
              n42 = Compound Arithmetic op=AND(w1945, w1943) -> (w1946:bool)
              n43 = local read "X Reference Time Period (uSec)"() -> (w1947:u32)
              n44 = case shown="True" w1946 {
                tunnel: [Control_X_Up_Down_Ramp."X Down Ramp" Control_X_Up_Down_Ramp."X Up Ramp"] -> w1942
                frame False {
                }
                frame True {
                }
              }
              n45 = local read "Fly Scan Running"() -> (w1941:bool)
              n46 = case shown="False" w1941 {
                tunnel: w1942 -> [_ w1972]
                tunnel: w1947 -> [_ w1971]
                tunnel: ["X Start Marker (nm)" w1970] -> w1940
                tunnel: w1948 -> [_ w1969]
                tunnel: w1955 -> [_ w1968]
                tunnel: w1937 -> [_ w1967]
                tunnel: w1938 -> [_ w1966]
                tunnel: [_ w1965] -> w1952
                tunnel: [_ w1964] -> w1951
                tunnel: w1950 -> [_ w1963]
                tunnel: w1949 -> [_ w1962]
                frame False {
                  n47 = local write "Next Do Down Ramp"(FALSE ("Restart Up Ramp")) -> ()
                  n48 = local write "Y Ramp Drop"(FALSE ("Y Toggle 1")) -> ()
                  "X scan done" <- TRUE
                }
                frame True {
                  n49 = case shown="\"X Down Ramp\"" w1972 {
                    tunnel: [w1991 _] -> w1965
                    tunnel: w1963 -> [w1990 _]
                    tunnel: w1971 -> [w1987 w2012]
                    tunnel: w1969 -> [w1986 w2008]
                    tunnel: w1967 -> [w1977 w1999]
                    tunnel: w1966 -> [w1975 w2000]
                    tunnel: [_ w2015] -> w1964
                    tunnel: w1962 -> [_ w2014]
                    tunnel: w1968 -> [w1982 w2006]
                    tunnel: [w1979 w2002] -> w1970
                    frame "X Up Ramp", Default {
                      n50 = Increment(x=w1990) -> (x+1=w1988:u32)
                      n51 = Multiply(x=w1988, y=w1987) -> (x*y=w1983:u32)
                      n52 = Multiply(x=w1983, y=w1982) -> (x*y=w1981:fxp<+,64,48>)
                      n53 = Less Or Equal?(x=w1983, y=w1986) -> (x <= y?=w1985:bool)
                      "X Ramp Mid Range" <- w1985
                      n54 = Add(x=w1981, y=w1977) -> (x+y=w1980:fxp<+/-,64,50>)
                      n55 = Greater?(x=w1983, y=w1986) -> (0:w1976:bool)
                      "If True End X Up Ramp" <- w1976
                      n56 = local write "Y Ramp Drop"(FALSE ("Y Ramp Drop")) -> ()
                      n57 = case shown="True" w1976 {
                        frame False {
                        }
                        frame True {
                          n58 = local write "Start or middle"(TRUE ("Start or middle")) -> ()
                          n59 = local write "Fly Scan"(FALSE ("Fly Scan Start")) -> ()
                          "Y Ramp Drop" <- TRUE ("Boolean")
                          "Next Do Down Ramp" <- TRUE
                        }
                      }
                      n60 = Greater?(x=w1980, y=w1975) -> (0:w1978:bool)
                      n61 = Select(t=w1988, s=w1985, f=u32 0) -> (s? t:f=w1989:u32)
                      n62 = Select(t=w1975, s=w1978, f=w1980) -> (s? t:f=w1979:fxp<+/-,64,50>)
                      n63 = Select(t=u32 0, s=w1976, f=w1989) -> (s? t:f=w1991:u32)
                      "Continue Run" <- TRUE ("Fly Scan Running")
                    }
                    frame "X Down Ramp" {
                      n64 = Increment(x=w2014) -> (x+1=w2013:u32)
                      n65 = Multiply(x=w2013, y=w2012) -> (x*y=w2007:u32)
                      n66 = Multiply(x=w2007, y=w2006) -> (x*y=w2005:fxp<+,64,48>)
                      n67 = Less Or Equal?(x=w2007, y=w2008) -> (x <= y?=w2011:bool)
                      n68 = Greater?(x=w2007, y=w2008) -> (0:w2001:bool)
                      "If True End X Down Ramp" <- w2001
                      n69 = local write "Y Ramp Drop"(FALSE ("Y Ramp Drop")) -> ()
                      n70 = Subtract(x=w2000, y=w2005) -> (x-y=w2003:fxp<+/-,64,50>)
                      n71 = case shown="True" w2001 {
                        frame False {
                        }
                        frame True {
                          n72 = local write "Y Ramp Drop"(TRUE ("Start Scan")) -> ()
                          n73 = local write "Start or middle"(TRUE ("Start or middle")) -> ()
                          n74 = local write "Next Do Down Ramp"(FALSE ("Next Do Down Ramp")) -> ()
                          n75 = local write "Fly Scan"(FALSE ("Fly Scan Start")) -> ()
                        }
                      }
                      n76 = Less?(x=w2003, y=w1999) -> (x < y?=w2004:bool)
                      n77 = Select(t=w2013, s=w2011, f=u32 0) -> (s? t:f=w2009:u32)
                      n78 = local write "Continue Run"(TRUE ("Fly Scan Running")) -> ()
                      n79 = Select(t=w1999, s=w2004, f=w2003) -> (s? t:f=w2002:fxp<+/-,64,50>)
                      n80 = Select(t=u32 0, s=w2001, f=w2009) -> (s? t:f=w2015:u32)
                    }
                  }
                }
              }
              n81 = To Fixed-Point(fixed-point type=fxp<+/-,58,25> 0.0, number=w1940) -> (fixed-point=w1939:fxp<+/-,58,25>)
            }
            frame "Filtered White Noise" {
              n82 = call "White Noise Generator"("seed"=w2033, "reset"=w2031, "amplitude"=w2030) -> ("white noise out"=w2032:i16)  [unwired: 12 in]
              n83 = xnode "Butterworth Filter"("input data"=w2032, "reset"=w2031) -> ("output data"=w2028:i16)  [unwired: 1 in]
              n84 = Divide(x=w2028, y=i16 32767) -> (x/y=w2023:fxp<+/-,41,18>)
              n85 = Multiply(x=w2023, y=w2021) -> (x*y=w2026:fxp<+/-,64,35>)
              n86 = Add(x=w2026, y=w2022) -> (x+y=w2025:fxp<+/-,64,36>)
              n87 = To Fixed-Point(fixed-point type=fxp<+/-,58,25> 0.0, number=w2025) -> (fixed-point=w2024:fxp<+/-,58,25>)
            }
          }
          "X Stage Reference (nm)" <- w1906
          n88 = call "measure_loop_rate_FPGA.vi"() -> ("Loop Rate (Ticks)"=→"Measured X Reference Time Period (Ticks)":u32)  [unwired: 11 in]
          n89 = local read "stop case"() -> (w1913:bool)
          n90 = call "Loop Timer"("Count(uSec)"="X Reference Time Period (uSec)") -> ()  [unwired: 1 out]
        }
        n91 = while {
          shift-right: [w397] -> _
          shift-left: i16 0 -> [w396]
          shift-right: [w395] -> _
          shift-left: i16 0 -> [w394]
          stop <- w407 stop-if-true
          n92 = local read "Fly Scan Running"() -> (w386:bool)
          n93 = case shown="\"Square Wave 1\"" "Trigger Wave Generator" {
            tunnel: [w423 w467 w489] -> w398
            tunnel: [w421 _ _] -> w397
            tunnel: w396 -> [w420 _ _]
            tunnel: [w414 _ _] -> w395
            tunnel: w394 -> [w413 _ _]
            tunnel: "DT Reset" -> [_ w473 w494]
            tunnel: "DT Frequency (periods/tick)" -> [_ w472 w493]
            tunnel: "DT Phase Offset (periods)" -> [_ w471 w492]
            tunnel: "DT Duty Cycle (periods)" -> [_ w470 _]
            tunnel: "DT Reference Amplitude (V)" -> [_ w469 w491]
            tunnel: "DT Reference DC Offset (V)" -> [_ w468 w490]
            tunnel: w386 -> [w408 w466 w488]
            frame "Custom Square Wave ", Default {
              n94 = local read "If True End Trigger High"() -> (w412:bool)
              n95 = local read "If True End Trigger Low"() -> (w411:bool)
              n96 = Not(x=w412) -> (.not. x?=w410:bool)
              n97 = Compound Arithmetic op=AND(w411, w410) -> (w409:bool)
              n98 = local read "Trigger Generation Time Period (uSec)"() -> (w419:u32)
              n99 = case shown="True" w409 {
                tunnel: [Detector_Trigger_Control."Trigger Low" Detector_Trigger_Control."Trigger High"] -> w422
                frame False {
                }
                frame True {
                }
              }
              n100 = case shown="True" w408 {
                tunnel: [fxp<+/-,20,5> 0.0 ("Trigger High Level (V)") w429] -> w423
                tunnel: w422 -> [_ w437]
                tunnel: [_ w436] -> w421
                tunnel: w420 -> [_ w435]
                tunnel: w419 -> [_ w434]
                tunnel: "Trigger High Period (usec)" -> [_ w433]
                tunnel: "Trigger Low Period (usec)" -> [_ w432]
                tunnel: "Trigger High Level (V)" -> [_ w431]
                tunnel: "Trigger Low Level (V)" -> [_ w430]
                tunnel: [_ w428] -> w414
                tunnel: w413 -> [_ w427]
                frame False {
                  n101 = local write "If True End Trigger High"(FALSE ("If True End Trigger High")) -> ()
                  n102 = local write "If True End Trigger Low"(TRUE ("If True End Trigger Low")) -> ()
                }
                frame True {
                  n103 = case shown="\"Trigger High\", Default" w437 {
                    tunnel: [w448 _] -> w436
                    tunnel: w435 -> [w447 _]
                    tunnel: w434 -> [w444 w458]
                    tunnel: w433 -> [w442 _]
                    tunnel: w432 -> [_ w456]
                    tunnel: w431 -> [w439 _]
                    tunnel: w430 -> [_ w451]
                    tunnel: [w439 w451] -> w429
                    tunnel: [_ w461] -> w428
                    tunnel: w427 -> [_ w460]
                    frame "Trigger High", Default {
                      n104 = Increment(x=w447) -> (x+1=w445:i16)
                      n105 = Multiply(x=w445, y=w444) -> (x*y=w443:u32)
                      n106 = Less Or Equal?(x=w443, y=w442) -> (x <= y?=w441:bool)
                      "Trigger Mid High" <- w441
                      n107 = Greater?(x=w443, y=w442) -> (0:w438:bool)
                      "If True End Trigger High" <- w438
                      n108 = case shown="True" w438 {
                        frame False {
                        }
                        frame True {
                          n109 = local write "If True End Trigger Low"(FALSE) -> ()
                        }
                      }
                      n110 = Select(t=w445, s=w441, f=i16 0) -> (s? t:f=w446:i16)
                      n111 = Select(t=i16 0, s=w438, f=w446) -> (s? t:f=w448:i16)
                    }
                    frame "Trigger Low" {
                      n112 = Increment(x=w460) -> (x+1=w459:i16)
                      n113 = Multiply(x=w459, y=w458) -> (x*y=w457:u32)
                      n114 = Less Or Equal?(x=w457, y=w456) -> (x <= y?=w455:bool)
                      n115 = Greater?(x=w457, y=w456) -> (0:w452:bool)
                      "If True End Trigger Low" <- w452
                      n116 = case shown="True" w452 {
                        frame False {
                        }
                        frame True {
                          n117 = local write "If True End Trigger High"(FALSE) -> ()
                        }
                      }
                      n118 = Select(t=w459, s=w455, f=i16 0) -> (s? t:f=w453:i16)
                      n119 = Select(t=i16 0, s=w452, f=w453) -> (s? t:f=w461:i16)
                    }
                  }
                }
              }
            }
            frame "Square Wave 1" {
              n120 = case shown="True" w466 {
                tunnel: w473 -> [_ w481]
                tunnel: w472 -> [_ w480]
                tunnel: w471 -> [_ w479]
                tunnel: w470 -> [_ w478]
                tunnel: w469 -> [_ w477]
                tunnel: w468 -> [_ w476]
                tunnel: [fxp<+/-,58,25> 0.0 ("fixed-point type") w475] -> w467
                frame False {
                }
                frame True {
                  n121 = call "Square Wave Generator"("frequency (periods/tick)"=w480, "reset"=w481, "phase offset (periods)"=w479, "duty cycle (periods)"=w478) -> ("square wave out"=w487:i16)  [unwired: 11 in]
                  n122 = Divide(x=w487, y=i16 32767) -> (x/y=w485:fxp<+/-,41,18>)
                  n123 = Multiply(x=w485, y=w477) -> (x*y=w484:fxp<+/-,64,35>)
                  n124 = Add(x=w484, y=w476) -> (x+y=w483:fxp<+/-,64,36>)
                  n125 = To Fixed-Point(fixed-point type=fxp<+/-,58,25> 0.0, number=w483) -> (fixed-point=w475:fxp<+/-,58,25>)
                }
              }
            }
            frame "Square Wave 2" {
              n126 = case shown="True" w488 {
                tunnel: w493 -> [_ w501]
                tunnel: w492 -> [_ w500]
                tunnel: w494 -> [_ w499]
                tunnel: w491 -> [_ w498]
                tunnel: w490 -> [_ w497]
                tunnel: [fxp<+/-,58,25> 0.0 ("fixed-point type") w496] -> w489
                frame False {
                }
                frame True {
                  w507 = fxp<+/-,32,16> 0.0 ("fixed-point type")
                  n127 = call "Sine Wave Generator3"("frequency (periods/tick)"=w501, "reset"=w499, "phase offset (periods)"=w500) -> ("sine out"=w506:i16)  [unwired: 12 in]
                  n128 = Divide(x=w506, y=i16 32767) -> (x/y=w527:fxp<+/-,41,18>)
                  n129 = Greater?(x=w527, y=w507) -> (0:w514:bool)
                  n130 = Equal?(x=w527, y=w507) -> (x = y?=w515:bool)
                  n131 = Less?(x=w527, y=w507) -> (x < y?=w513:bool)
                  n132 = Not(x=w514) -> (.not. x?=w511:bool)
                  n133 = Not(x=w515) -> (.not. x?=w510:bool)
                  n134 = Not(x=w513) -> (.not. x?=w512:bool)
                  n135 = Compound Arithmetic op=AND(w514, w510, w512) -> (w516:bool)
                  n136 = Compound Arithmetic op=AND(w511, w515, w512) -> (w509:bool)
                  n137 = Compound Arithmetic op=AND(w511, w510, w513) -> (w508:bool)
                  n138 = Select(t=fxp<+/-,2,2> 1.0 ("fixed-point type"), s=w516, f=fxp<+/-,2,2> 0.0 ("fixed-point type")) -> (s? t:f=w520:fxp<+/-,2,2>)
                  n139 = Select(t=fxp<+/-,2,2> 0.0 ("fixed-point type"), s=w509, f=fxp<+/-,2,2> 0.0 ("fixed-point type")) -> (s? t:f=w519:fxp<+/-,2,2>)
                  n140 = Select(t=fxp<+/-,2,2> -1.0 ("fixed-point type"), s=w508, f=fxp<+/-,2,2> 0.0 ("fixed-point type")) -> (s? t:f=w517:fxp<+/-,2,2>)
                  n141 = Add(x=w520, y=w519) -> (x+y=w518:fxp<+/-,3,3>)
                  n142 = Add(x=w518, y=w517) -> (x+y=w503:fxp<+/-,4,4>)
                  n143 = Multiply(x=w503, y=w498) -> (x*y=w504:fxp<+/-,43,20>)
                  n144 = Add(x=w504, y=w497) -> (x+y=w502:fxp<+/-,43,20>)
                  n145 = To Fixed-Point(fixed-point type=fxp<+/-,58,25> 0.0, number=w502) -> (fixed-point=w496:fxp<+/-,58,25>)
                }
              }
            }
          }
          n146 = call "measure_loop_rate_FPGA.vi"() -> ("Loop Rate (Ticks)"=→"Measured Trigger Gen Time Period (Ticks)":u32)  [unwired: 11 in]
          n147 = To Fixed-Point(fixed-point type=fxp<+/-,20,5> 0.0, number=w398) -> (fixed-point=w399:fxp<+/-,20,5>)
          n148 = In Range and Coerce(upper limit="Detector Trigger Upper Limit (V)", x=w399, lower limit="Detector Trigger Lower Limit (V)") -> (coerced(x)=→"Detector Trigger (V)":fxp<+/-,20,5>, In Range?=→"Detector Trigger In Range?":bool)
          n149 = call "Loop Timer7"("Count(uSec)"="Trigger Generation Time Period (uSec)") -> ()  [unwired: 1 out]
          n150 = local read "stop case"() -> (w407:bool)
        }
        n151 = while {
          stop <- w135 stop-if-true
          n152 = call "measure_loop_rate_FPGA.vi"() -> ("Loop Rate (Ticks)"=→"Measured Z Reference Time Period (Ticks)":u32)  [unwired: 11 in]
          n153 = call "Loop Timer10"("Count(uSec)"="Z Reference Time Period (uSec)") -> ()  [unwired: 1 out]
          n154 = case shown="\"Filtered White Noise\"" "Z Reference Wave Selection" {
            tunnel: "Z Reference Reset" -> [_ w165 w172 w188 w221]
            tunnel: "Z Frequency (periods/tick)" -> [_ w164 w171 w187 _]
            tunnel: "Z Phase Offset (periods)" -> [_ w163 w170 w186 _]
            tunnel: "Z White Noise Seed" -> [_ _ _ _ w223]
            tunnel: "Z White Noise Amplitude" -> [_ _ _ _ w222]
            tunnel: "Z Reference DC Offset (nm)" -> [w147 w156 w167 w178 w212]
            tunnel: "Z Reference Amplitude (nm)" -> [w148 w157 w166 w180 w213]
            tunnel: [w149 w154 w168 w183 w211] -> w136
            frame "Constant", Default {
              n155 = Multiply(x=i16 1 ("y"), y=w148) -> (x*y=w152:fxp<+/-,56,33>)
              n156 = Add(x=w152, y=w147) -> (x+y=w151:fxp<+/-,56,33>)
              n157 = To Fixed-Point(fixed-point type=fxp<+/-,58,25> 0.0, number=w151) -> (fixed-point=w149:fxp<+/-,58,25>)
            }
            frame "Sine Wave" {
              n158 = call "Sine Wave Generator2"("frequency (periods/tick)"=w164, "reset"=w165, "phase offset (periods)"=w163) -> ("sine out"=w158:i16)  [unwired: 12 in]
              n159 = Divide(x=w158, y=i16 32767) -> (x/y=w161:fxp<+/-,41,18>)
              n160 = Multiply(x=w161, y=w157) -> (x*y=w160:fxp<+/-,64,35>)
              n161 = Add(x=w160, y=w156) -> (x+y=w159:fxp<+/-,64,36>)
              n162 = To Fixed-Point(fixed-point type=fxp<+/-,58,25> 0.0, number=w159) -> (fixed-point=w154:fxp<+/-,58,25>)
            }
            frame "Sawtooth Wave" {
              n163 = call "Saw Wave Generator.vi"("frequency (periods/tick)"=w171, "reset"=w172, "phase offset (periods)"=w170) -> ("saw out"=w169:i16)  [unwired: 12 in]
              n164 = Divide(x=w169, y=i16 32767) -> (x/y=w176:fxp<+/-,41,18>)
              n165 = Multiply(x=w176, y=w166) -> (x*y=w175:fxp<+/-,64,35>)
              n166 = Add(x=w175, y=w167) -> (x+y=w174:fxp<+/-,64,36>)
              n167 = To Fixed-Point(fixed-point type=fxp<+/-,58,25> 0.0, number=w174) -> (fixed-point=w168:fxp<+/-,58,25>)
            }
            frame "Square Wave" {
              w189 = fxp<+/-,32,16> 0.0 ("fixed-point type")
              n168 = call "Sine Wave Generator5"("frequency (periods/tick)"=w187, "reset"=w188, "phase offset (periods)"=w186) -> ("sine out"=w185:i16)  [unwired: 12 in]
              n169 = Divide(x=w185, y=i16 32767) -> (x/y=w209:fxp<+/-,41,18>)
              n170 = Greater?(x=w209, y=w189) -> (0:w196:bool)
              n171 = Less?(x=w209, y=w189) -> (x < y?=w195:bool)
              n172 = Equal?(x=w209, y=w189) -> (x = y?=w197:bool)
              n173 = Not(x=w196) -> (.not. x?=w193:bool)
              n174 = Not(x=w195) -> (.not. x?=w194:bool)
              n175 = Not(x=w197) -> (.not. x?=w192:bool)
              n176 = Compound Arithmetic op=AND(w196, w192, w194) -> (w198:bool)
              n177 = Compound Arithmetic op=AND(w193, w197, w194) -> (w191:bool)
              n178 = Compound Arithmetic op=AND(w193, w192, w195) -> (w190:bool)
              n179 = Select(t=fxp<+/-,2,2> 1.0 ("fixed-point type"), s=w198, f=fxp<+/-,2,2> 0.0 ("fixed-point type")) -> (s? t:f=w202:fxp<+/-,2,2>)
              n180 = Select(t=fxp<+/-,2,2> 0.0 ("fixed-point type"), s=w191, f=fxp<+/-,2,2> 0.0 ("fixed-point type")) -> (s? t:f=w201:fxp<+/-,2,2>)
              n181 = Add(x=w202, y=w201) -> (x+y=w200:fxp<+/-,3,3>)
              n182 = Select(t=fxp<+/-,2,2> -1.0 ("fixed-point type"), s=w190, f=fxp<+/-,2,2> 0.0 ("fixed-point type")) -> (s? t:f=w199:fxp<+/-,2,2>)
              n183 = Add(x=w200, y=w199) -> (x+y=w181:fxp<+/-,4,4>)
              n184 = Multiply(x=w181, y=w180) -> (x*y=w182:fxp<+/-,43,20>)
              n185 = Add(x=w182, y=w178) -> (x+y=w179:fxp<+/-,43,20>)
              n186 = To Fixed-Point(fixed-point type=fxp<+/-,58,25> 0.0, number=w179) -> (fixed-point=w183:fxp<+/-,58,25>)
            }
            frame "Filtered White Noise" {
              n187 = call "White Noise Generator3"("seed"=w223, "reset"=w221, "amplitude"=w222) -> ("white noise out"=w220:i16)  [unwired: 12 in]
              n188 = xnode "Butterworth Filter"("input data"=w220, "reset"=w221) -> ("output data"=w215:i16)  [unwired: 1 in]
              n189 = Divide(x=w215, y=i16 32767) -> (x/y=w218:fxp<+/-,41,18>)
              n190 = Multiply(x=w218, y=w213) -> (x*y=w217:fxp<+/-,64,35>)
              n191 = Add(x=w217, y=w212) -> (x+y=w216:fxp<+/-,64,36>)
              n192 = To Fixed-Point(fixed-point type=fxp<+/-,58,25> 0.0, number=w216) -> (fixed-point=w211:fxp<+/-,58,25>)
            }
          }
          "Z Stage Reference (nm)" <- w136
          n193 = local read "stop case"() -> (w135:bool)
        }
        n194 = while {
          shift-right: [w240] -> _
          shift-left: _ -> [w235]
          shift-right: [w239] -> _
          shift-left: u32 0 ("f") -> [w237]
          shift-right: [w238] -> _
          shift-left: u32 0 -> [w236]
          stop <- w241 stop-if-true
          n195 = case shown="\"Custom Ramp Wave\"" "Y Reference Wave Selection" {
            tunnel: "Y Reference Amplitude (nm)" -> [w258 w262 _ w363]
            tunnel: "Y Reference DC Offset (nm)" -> [w257 w261 _ w362]
            tunnel: [w253 w260 w288 w359] -> w249
            tunnel: "Y Frequency (periods/tick)" -> [_ w271 _ _]
            tunnel: "Y Phase Offset (periods)" -> [_ w270 _ _]
            tunnel: "Y Reference Reset" -> [_ w269 _ w368]
            tunnel: "Y White Noise Seed" -> [_ _ _ w371]
            tunnel: "Y White Noise Amplitude" -> [_ _ _ w370]
            tunnel: [_ _ w286 _] -> w240
            tunnel: [_ _ w284 _] -> w239
            tunnel: [_ _ w283 _] -> w238
            tunnel: w237 -> [_ _ w282 _]
            tunnel: w236 -> [_ _ w281 _]
            tunnel: w235 -> [_ _ w279 _]
            tunnel: "Y Ramp Period (usec)" -> [_ _ w275 _]
            tunnel: "Y Ramp End (nm)" -> [_ _ w274 _]
            tunnel: "Y Ramp Start (nm)" -> [_ _ w273 _]
            frame "Constant", Default {
              n196 = Multiply(x=i16 1 ("y"), y=w258) -> (x*y=w256:fxp<+/-,56,33>)
              n197 = Add(x=w256, y=w257) -> (x+y=w255:fxp<+/-,56,33>)
              n198 = To Fixed-Point(fixed-point type=fxp<+/-,58,25> 0.0, number=w255) -> (fixed-point=w253:fxp<+/-,58,25>)
            }
            frame "Sine Wave" {
              n199 = call "Sine Wave Generator4"("frequency (periods/tick)"=w271, "reset"=w269, "phase offset (periods)"=w270) -> ("sine out"=w268:i16)  [unwired: 12 in]
              n200 = Divide(x=w268, y=i16 32767) -> (x/y=w266:fxp<+/-,41,18>)
              n201 = Multiply(x=w266, y=w262) -> (x*y=w265:fxp<+/-,64,35>)
              n202 = Add(x=w265, y=w261) -> (x+y=w264:fxp<+/-,64,36>)
              n203 = To Fixed-Point(fixed-point type=fxp<+/-,58,25> 0.0, number=w264) -> (fixed-point=w260:fxp<+/-,58,25>)
            }
            frame "Custom Ramp Wave" {
              n204 = Subtract(x=w273, y=w274) -> (x-y=w293:fxp<+/-,17,17>)
              n205 = Less?(x=w273, y=w274) -> (x < y?=w278:bool)
              n206 = Absolute Value(x=w293) -> (abs(x)=w292:fxp<+,16,16>)
              n207 = local read "Continue Run"() -> (w277:bool)
              n208 = Divide(x=w292, y=w275) -> (x/y=w294:fxp<+,48,16>)
              "Y Ramp Slope" <- w294
              n209 = local read "Start or middle"() -> (w290:bool)
              n210 = local read "Y Reference Time Period (uSec)"() -> (w280:u32)
              n211 = case shown="True" w278 {
                tunnel: [Control_Y_Up_Down_Ramp."Y Down Ramp" Control_Y_Up_Down_Ramp."Y Up Ramp"] -> w276
                frame False {
                }
                frame True {
                }
              }
              n212 = Compound Arithmetic op=OR("Fly Scan", w277) -> (w285:bool)
              "Fly Scan Running" <- w285
              n213 = Select(t=w279, s=w290, f=w273) -> (s? t:f=w291:fxp<+/-,58,25>)
              n214 = case shown="False" w285 {
                tunnel: w276 -> [_ w312]
                tunnel: w280 -> [_ w311]
                tunnel: ["Y Start Marker (nm)" w310] -> w289
                tunnel: w275 -> [_ w309]
                tunnel: w294 -> [_ w308]
                tunnel: w273 -> [_ w307]
                tunnel: w274 -> [_ w306]
                tunnel: [_ w305] -> w284
                tunnel: [_ w304] -> w283
                tunnel: w282 -> [_ w303]
                tunnel: w281 -> [_ w302]
                tunnel: [_ w301] -> w286
                tunnel: w291 -> [_ w300]
                frame False {
                  "Start or middle" <- FALSE ("Start or middle")
                  "Y scan done" <- TRUE
                }
                frame True {
                  n215 = case shown="\"Y Down Ramp\"" w312 {
                    tunnel: [w331 _] -> w305
                    tunnel: w303 -> [w330 _]
                    tunnel: w311 -> [w327 w348]
                    tunnel: w309 -> [w326 w344]
                    tunnel: w307 -> [w316 _]
                    tunnel: w306 -> [w320 w337]
                    tunnel: [_ w351] -> w304
                    tunnel: w302 -> [_ w350]
                    tunnel: w308 -> [w322 _]
                    tunnel: [w314 w333] -> w310
                    tunnel: [_ w333] -> w301
                    tunnel: w300 -> [_ w335]
                    frame "Y Up Ramp", Default {
                      n216 = Increment(x=w330) -> (x+1=w328:u32)
                      n217 = Multiply(x=w328, y=w327) -> (x*y=w323:u32)
                      n218 = Multiply(x=w323, y=w322) -> (x*y=w321:fxp<+,64,48>)
                      n219 = Less Or Equal?(x=w323, y=w326) -> (x <= y?=w325:bool)
                      "Ramp Mid Range" <- w325
                      n220 = Add(x=w321, y=w316) -> (x+y=w319:fxp<+/-,64,50>)
                      n221 = Greater?(x=w323, y=w326) -> (0:w315:bool)
                      "If True End Up Ramp" <- w315
                      n222 = Greater?(x=w319, y=w320) -> (0:w317:bool)
                      n223 = Select(t=w328, s=w325, f=i16 0) -> (s? t:f=w329:u32)
                      n224 = Select(t=w316, s=w317, f=w319) -> (s? t:f=w318:fxp<+/-,64,50>)
                      n225 = Select(t=i16 0, s=w315, f=w329) -> (s? t:f=w331:u32)
                      n226 = To Fixed-Point(fixed-point type=fxp<+/-,58,25> 0.0, number=w318) -> (fixed-point=w314:fxp<+/-,58,25>)
                    }
                    frame "Y Down Ramp" {
                      n227 = Increment(x=w350) -> (x+1=w349:u32)
                      n228 = local read "Y Ramp Drop"() -> (w341:bool)
                      n229 = Multiply(x=w349, y=w348) -> (x*y=w343:u32)
                      n230 = Less Or Equal?(x=w343, y=w344) -> (x <= y?=w347:bool)
                      n231 = Greater?(x=w343, y=w344) -> (0:w342:bool)
                      "If True End Y Down Ramp" <- w342
                      n232 = case shown="False" w341 {
                        tunnel: "Y Ramp Drop Size (nm)" -> [_ w356]
                        tunnel: [w353 w355] -> w339
                        tunnel: w335 -> [w353 w354]
                        frame False {
                        }
                        frame True {
                          n233 = Subtract(x=w354, y=w356) -> (x-y=w355:fxp<+/-,59,26>)
                        }
                      }
                      n234 = Select(t=w349, s=w347, f=u32 0) -> (s? t:f=w345:u32)
                      n235 = To Fixed-Point(fixed-point type=fxp<+/-,58,25> 0.0, number=w339) -> (fixed-point=w334:fxp<+/-,58,25>)
                      n236 = Less?(x=w334, y=w337) -> (x < y?=w336:bool)
                      n237 = case shown="True" w336 {
                        frame False {
                        }
                        frame True {
                          n238 = local write "Fly Scan Running"(FALSE ("Fly Scan Running")) -> ()
                          n239 = local write "Continue Run"(FALSE ("Start Scan")) -> ()
                        }
                      }
                      n240 = Select(t=u32 0, s=w342, f=w345) -> (s? t:f=w351:u32)
                      n241 = Select(t=w335, s=w336, f=w334) -> (s? t:f=w333:fxp<+/-,58,25>)
                    }
                  }
                }
              }
              n242 = To Fixed-Point(fixed-point type=fxp<+/-,58,25> 0.0, number=w289) -> (fixed-point=w288:fxp<+/-,58,25>)
            }
            frame "Filtered White Noise" {
              n243 = call "White Noise Generator2"("seed"=w371, "reset"=w368, "amplitude"=w370) -> ("white noise out"=w369:i16)  [unwired: 12 in]
              n244 = xnode "Butterworth Filter"("input data"=w369, "reset"=w368) -> ("output data"=w366:i16)  [unwired: 1 in]
              n245 = Divide(x=w366, y=i16 32767) -> (x/y=w365:fxp<+/-,41,18>)
              n246 = Multiply(x=w365, y=w363) -> (x*y=w364:fxp<+/-,64,35>)
              n247 = Add(x=w364, y=w362) -> (x+y=w361:fxp<+/-,64,36>)
              n248 = To Fixed-Point(fixed-point type=fxp<+/-,58,25> 0.0, number=w361) -> (fixed-point=w359:fxp<+/-,58,25>)
            }
          }
          "Y Stage Reference (nm)" <- w249
          n249 = call "measure_loop_rate_FPGA.vi"() -> ("Loop Rate (Ticks)"=→"Measured Y Reference Time Period (Ticks)":u32)  [unwired: 11 in]
          n250 = local read "stop case"() -> (w241:bool)
          n251 = call "Loop Timer9"("Count(uSec)"="Y Reference Time Period (uSec)") -> ()  [unwired: 1 out]
        }
        n252 = node-c288(refnum<k21> "40 MHz Onboard Clock" ("Source Name"), w111) -> (w119:T12)
        n253 = while {
          shift-right: [w782] -> _
          shift-left: _ -> [w773]
          shift-right: [w781] -> _
          shift-left: _ -> [w772]
          shift-right: [w780] -> _
          shift-left: _ -> [w771]
          shift-right: [w779] -> _
          shift-left: _ -> [w770]
          shift-right: [w778] -> _
          shift-left: _ -> [w769]
          shift-right: [w777] -> _
          shift-left: _ -> [w768]
          shift-right: [w776] -> _
          shift-left: _ -> [w767]
          shift-right: [w775] -> _
          shift-left: _ -> [w766]
          shift-right: [w774] -> _
          shift-left: _ -> [w765]
          shift-right: [w759] -> _
          shift-left: _ -> [w758]
          shift-right: [w757] -> _
          shift-left: _ -> [w756]
          shift-right: [w755] -> _
          shift-left: _ -> [w754]
          shift-right: [w753] -> _
          shift-left: _ -> [w752]
          shift-right: [w751] -> _
          shift-left: _ -> [w750]
          shift-right: [w749] -> _
          shift-left: _ -> [w748]
          shift-right: [w746] -> _
          shift-left: _ -> [w745]
          shift-right: [w747] -> _
          shift-left: _ -> [w744]
          shift-right: [w743] -> _
          shift-left: _ -> [w741]
          shift-right: [w742] -> _
          shift-left: _ -> [w740]
          shift-right: [w739] -> _
          shift-left: _ -> [w737]
          shift-right: [w738] -> _
          shift-left: _ -> [w736]
          shift-right: [w735] -> _
          shift-left: _ -> [w733]
          shift-right: [w734] -> _
          shift-left: _ -> [w732]
          shift-right: [w730] -> _
          shift-left: _ -> [w728]
          shift-right: [w731] -> _
          shift-left: _ -> [w729]
          shift-right: [w726] -> _
          shift-left: _ -> [w724]
          shift-right: [w727] -> _
          shift-left: _ -> [w725]
          stop <- w795 stop-if-true
          w760 = fxp<+/-,20,5> 0.0 ("fixed-point type")
          n254 = local read "Sample X Stage Displacement (nm)"() -> (w720:fxp<+/-,58,25>)
          n255 = local read "Sample Y Stage Displacement (nm)"() -> (w717:fxp<+/-,58,25>)
          n256 = local read "Sample Z Stage Displacement (nm)"() -> (w714:fxp<+/-,58,25>)
          n257 = local read "Optics Z Stage Displacement (nm)"() -> (w713:fxp<+/-,58,25>)
          n258 = local read "Optics X Stage Displacement (nm)"() -> (w719:fxp<+/-,58,25>)
          n259 = local read "Optics Y Stage Displacement (nm)"() -> (w716:fxp<+/-,58,25>)
          n260 = case shown="\"FPGA Generated Reference\", Default" "Reference Signal Source" {
            tunnel: [w799 w802] -> w723
            tunnel: [w798 w801] -> w722
            tunnel: [w797 w800] -> w721
            frame "FPGA Generated Reference", Default {
              n261 = local read "X Stage Reference (nm)"() -> (w799:fxp<+/-,58,25>)
              n262 = local read "Y Stage Reference (nm)"() -> (w798:fxp<+/-,58,25>)
              n263 = local read "Z Stage Reference (nm)"() -> (w797:fxp<+/-,58,25>)
            }
            frame "External Reference" {
              n264 = local read "X Stage External Reference (nm)"() -> (w802:fxp<+/-,58,25>)
              n265 = local read "Y Stage External Reference (nm)"() -> (w801:fxp<+/-,58,25>)
              n266 = local read "Z Stage External Reference (nm)"() -> (w800:fxp<+/-,58,25>)
            }
          }
          n267 = case shown="\"Optics Stage Only\", Default" "Optics and or Sample Stage" {
            tunnel: w720 -> [_ w814]
            tunnel: w719 -> [w805 w813]
            tunnel: [w805 w812] -> w718
            tunnel: w717 -> [_ w811]
            tunnel: w716 -> [w804 w810]
            tunnel: [w804 w809] -> w715
            tunnel: w714 -> [_ w808]
            tunnel: w713 -> [w803 w807]
            tunnel: [w803 w806] -> w712
            frame "Optics Stage Only", Default {
            }
            frame "Optics and Sample Stage" {
              n268 = Subtract(x=w813, y=w814) -> (x-y=w812:fxp<+/-,59,26>)
              n269 = Subtract(x=w810, y=w811) -> (x-y=w809:fxp<+/-,59,26>)
              n270 = Subtract(x=w807, y=w808) -> (x-y=w806:fxp<+/-,59,26>)
            }
          }
          n271 = call "Loop Timer3"("Count(uSec)"="Controller Time Period (uSec)") -> ()  [unwired: 1 out]
          n272 = case shown="\"Closed Loop\"" "System Loop Type" {
            tunnel: w718 -> [_ w918]
            tunnel: w723 -> [w830 w919]
            tunnel: [w823 w892] -> w784
            tunnel: [w824 w917] -> w764
            tunnel: [_ w914] -> w782
            tunnel: [_ w913] -> w781
            tunnel: [_ w912] -> w780
            tunnel: [_ w911] -> w779
            tunnel: [_ w910] -> w778
            tunnel: [_ w909] -> w777
            tunnel: [_ w908] -> w776
            tunnel: [_ w907] -> w775
            tunnel: [_ w906] -> w774
            tunnel: w772 -> [_ w905]
            tunnel: w771 -> [_ w904]
            tunnel: w770 -> [_ w903]
            tunnel: w769 -> [_ w902]
            tunnel: w768 -> [_ w901]
            tunnel: w767 -> [_ w900]
            tunnel: w766 -> [_ w899]
            tunnel: w765 -> [_ w898]
            tunnel: w715 -> [_ w896]
            tunnel: w722 -> [w829 w897]
            tunnel: w721 -> [w828 w890]
            tunnel: w712 -> [_ w889]
            tunnel: [w822 w893] -> w783
            tunnel: w773 -> [_ w895]
            tunnel: [_ w885] -> w759
            tunnel: w758 -> [_ w884]
            tunnel: [_ w883] -> w757
            tunnel: w756 -> [_ w882]
            tunnel: [_ w881] -> w755
            tunnel: w754 -> [_ w880]
            tunnel: [_ w874] -> w753
            tunnel: w752 -> [_ w873]
            tunnel: [_ w872] -> w751
            tunnel: w750 -> [_ w871]
            tunnel: [_ w870] -> w749
            tunnel: w748 -> [_ w869]
            tunnel: [_ w863] -> w746
            tunnel: [_ w862] -> w747
            tunnel: w745 -> [_ w861]
            tunnel: w744 -> [_ w860]
            tunnel: [_ w859] -> w743
            tunnel: [_ w858] -> w742
            tunnel: w741 -> [_ w857]
            tunnel: w740 -> [_ w856]
            tunnel: [_ w855] -> w739
            tunnel: [_ w854] -> w738
            tunnel: w737 -> [_ w853]
            tunnel: w736 -> [_ w852]
            tunnel: [_ w851] -> w735
            tunnel: [_ w850] -> w734
            tunnel: w733 -> [_ w849]
            tunnel: w732 -> [_ w848]
            tunnel: [_ w842] -> w731
            tunnel: [_ w841] -> w730
            tunnel: w729 -> [_ w840]
            tunnel: w728 -> [_ w839]
            tunnel: [_ w838] -> w727
            tunnel: [_ w837] -> w726
            tunnel: w725 -> [_ w836]
            tunnel: w724 -> [_ w835]
            frame "Open Loop", Default {
              w821 = fxp<+/-,58,25> 0.0 ("fixed-point type")
              n273 = Multiply(x="X-Stage nm to V Scaling", y="X-Stage Scaling Direction") -> (x*y=w832:fxp<+/-,35,15>)
              n274 = Multiply(x="Y-Stage nm to V Scaling", y="Y-Stage Scaling Direction") -> (x*y=w818:fxp<+/-,35,15>)
              n275 = Multiply(x="Z-Stage nm to V Scaling", y="Z-Stage Scaling Direction") -> (x*y=w817:fxp<+/-,35,15>)
              n276 = Multiply(x=w830, y=w832) -> (x*y=w827:fxp<+/-,64,38>)
              n277 = Multiply(x=w829, y=w818) -> (x*y=w826:fxp<+/-,64,38>)
              n278 = Multiply(x=w828, y=w817) -> (x*y=w825:fxp<+/-,64,38>)
              n279 = To Fixed-Point(fixed-point type=w821, number=w827) -> (fixed-point=w824:fxp<+/-,58,25>)
              n280 = To Fixed-Point(fixed-point type=w821, number=w826) -> (fixed-point=w823:fxp<+/-,58,25>)
              n281 = To Fixed-Point(fixed-point type=w821, number=w825) -> (fixed-point=w822:fxp<+/-,58,25>)
            }
            frame "Closed Loop" {
              w834 = fxp<+/-,58,25> 0.0 ("fixed-point type")
              w886 = fxp<+/-,58,25> 0.0 ("fixed-point type")
              n282 = Subtract(x=w919, y=w918) -> (x-y=w923:fxp<+/-,60,27>)
              n283 = Subtract(x=w897, y=w896) -> (x-y=w922:fxp<+/-,60,27>)
              n284 = Subtract(x=w890, y=w889) -> (x-y=w891:fxp<+/-,60,27>)
              n285 = To Fixed-Point(fixed-point type=w834, number=w923) -> (fixed-point=w921:fxp<+/-,58,25>)
              n286 = To Fixed-Point(fixed-point type=w834, number=w922) -> (fixed-point=w920:fxp<+/-,58,25>)
              n287 = To Fixed-Point(fixed-point type=w834, number=w891) -> (fixed-point=w888:fxp<+/-,58,25>)
              n288 = for {
                N: 9 -> [_]
                shift-right: [w1158] -> w876
                shift-left: _ -> [w1156]
                shift-right: [w1155] -> w866
                shift-left: _ -> [w1153]
                tunnel: [w1146] -> w914
                shift-right: [w1145] -> _
                shift-left: _ -> [w1141]
                tunnel: [w1144] -> w913
                shift-right: [w1143] -> _
                shift-left: _ -> [w1139]
                tunnel: w895 -> [w1136]
                tunnel: w905 -> [w1135]
                tunnel: [w1134] -> w911
                shift-right: [w1133] -> _
                shift-left: _ -> [w1126]
                tunnel: [w1132] -> w910
                shift-right: [w1131] -> _
                shift-left: _ -> [w1125]
                tunnel: [w1130] -> w908
                tunnel: [w1129] -> w907
                shift-right: [w1128] -> _
                shift-left: _ -> [w1124]
                shift-right: [w1127] -> _
                shift-left: _ -> [w1113]
                tunnel: w903 -> [w1123]
                tunnel: w902 -> [w1122]
                tunnel: w900 -> [w1121]
                tunnel: w899 -> [w1120]
                tunnel: w921 -> [w1112]
                tunnel: w920 -> [w1109]
                shift-right: [w1108] -> w846
                shift-left: _ -> [w1104]
                tunnel: [w1099] -> w912
                tunnel: [w1098] -> w909
                tunnel: [w1097] -> w906
                shift-right: [w1096] -> _
                shift-left: _ -> [w1092]
                shift-right: [w1095] -> _
                shift-left: _ -> [w1090]
                shift-right: [w1094] -> _
                shift-left: _ -> [w1088]
                tunnel: w904 -> [w1087]
                tunnel: w898 -> [w1086]
                tunnel: w901 -> [w1085]
                tunnel: w888 -> [w1081]
                shift-right: [w1078] -> w878
                shift-left: _ -> [w1076]
                tunnel: [w1074] -> w885
                shift-right: [w1075] -> _
                shift-left: _ -> [w1070]
                tunnel: w884 -> [w1069]
                tunnel: [w1066] -> w883
                shift-right: [w1065] -> _
                shift-left: _ -> [w1063]
                tunnel: w882 -> [w1064]
                tunnel: [w1059] -> w881
                shift-right: [w1058] -> _
                shift-left: _ -> [w1056]
                tunnel: w880 -> [w1055]
                shift-right: [w1054] -> w879
                shift-left: _ -> [w1051]
                tunnel: [w1047] -> w874
                shift-right: [w1048] -> _
                shift-left: _ -> [w1044]
                tunnel: w873 -> [w1046]
                tunnel: [w1041] -> w872
                shift-right: [w1040] -> _
                shift-left: _ -> [w1037]
                tunnel: w871 -> [w1039]
                tunnel: [w1034] -> w870
                shift-right: [w1033] -> _
                shift-left: _ -> [w1031]
                tunnel: w869 -> [w1030]
                shift-right: [w1026] -> w865
                shift-left: _ -> [w1023]
                shift-right: [w1025] -> w867
                shift-left: _ -> [w1021]
                tunnel: [w1016] -> w863
                shift-right: [w1015] -> _
                shift-left: _ -> [w1009]
                tunnel: [w1014] -> w862
                shift-right: [w1013] -> _
                shift-left: _ -> [w1007]
                tunnel: w861 -> [w1006]
                tunnel: w860 -> [w1005]
                tunnel: [w1003] -> w859
                shift-right: [w1002] -> _
                shift-left: _ -> [w995]
                tunnel: [w999] -> w858
                shift-right: [w998] -> _
                shift-left: _ -> [w993]
                tunnel: w857 -> [w992]
                tunnel: w856 -> [w991]
                tunnel: [w988] -> w855
                tunnel: [w986] -> w854
                shift-right: [w987] -> _
                shift-left: _ -> [w979]
                shift-right: [w985] -> _
                shift-left: _ -> [w981]
                tunnel: w853 -> [w978]
                tunnel: w852 -> [w977]
                tunnel: [w972] -> w851
                tunnel: [w971] -> w850
                shift-right: [w970] -> _
                shift-left: _ -> [w967]
                shift-right: [w969] -> _
                shift-left: _ -> [w965]
                tunnel: w849 -> [w964]
                tunnel: w848 -> [w963]
                shift-right: [w960] -> w844
                shift-left: _ -> [w957]
                shift-right: [w959] -> w845
                shift-left: _ -> [w955]
                tunnel: [w950] -> w842
                tunnel: [w949] -> w841
                shift-right: [w948] -> _
                shift-left: _ -> [w943]
                shift-right: [w947] -> _
                shift-left: _ -> [w941]
                tunnel: w840 -> [w940]
                tunnel: w839 -> [w939]
                shift-right: [w934] -> _
                shift-left: _ -> [w929]
                shift-right: [w933] -> _
                shift-left: _ -> [w927]
                tunnel: [w932] -> w838
                tunnel: [w931] -> w837
                tunnel: w836 -> [w926]
                tunnel: w835 -> [w925]
                i -> [w1164]
                # "ez"
                # "ey"
                # "ex"
                n289 = Add(x=1, y=w1164) -> (x+y=w1161:i32)
                n290 = flat-sequence {
                  tunnel: [w1298] -> w1178
                  tunnel: [w1297] -> w1177
                  tunnel: [w1296] -> w1176
                  tunnel: [w1295] -> w1175
                  tunnel: [w1294] -> w1174
                  tunnel: [w1293] -> w1173
                  tunnel: [w1292] -> w1172
                  tunnel: [w1291] -> w1171
                  tunnel: w1161 -> [w1299]
                  tunnel: [w1277] -> w1166
                  tunnel: [w1290] -> w1157
                  tunnel: w1156 -> [w1290]
                  tunnel: [w1289] -> w1154
                  tunnel: w1153 -> [w1289]
                  tunnel: [w1288] -> w1142
                  tunnel: w1141 -> [w1288]
                  tunnel: [w1215] -> w1140
                  tunnel: w1139 -> [w1215]
                  tunnel: w1136 -> [w1279]
                  tunnel: w1135 -> [w1280]
                  tunnel: w1126 -> [w1287]
                  tunnel: w1125 -> [w1286]
                  tunnel: w1124 -> [w1285]
                  tunnel: w1123 -> [w1281]
                  tunnel: w1122 -> [w1282]
                  tunnel: w1121 -> [w1283]
                  tunnel: w1120 -> [w1284]
                  tunnel: w1113 -> [w1278]
                  tunnel: [w1287] -> w1119
                  tunnel: [w1286] -> w1118
                  tunnel: [w1285] -> w1117
                  tunnel: w1112 -> [w1253]
                  tunnel: [w1278] -> w1111
                  tunnel: w1109 -> [w1275]
                  tunnel: [w1276] -> w1105
                  tunnel: w1104 -> [w1276]
                  tunnel: [w1274] -> w1093
                  tunnel: w1092 -> [w1274]
                  tunnel: [w1273] -> w1091
                  tunnel: w1090 -> [w1273]
                  tunnel: [w1272] -> w1089
                  tunnel: w1088 -> [w1272]
                  tunnel: w1087 -> [w1269]
                  tunnel: w1086 -> [w1271]
                  tunnel: w1085 -> [w1270]
                  tunnel: w1081 -> [w1252]
                  tunnel: [w1246] -> w1077
                  tunnel: w1076 -> [w1246]
                  tunnel: [w1245] -> w1071
                  tunnel: w1070 -> [w1245]
                  tunnel: w1069 -> [w1244]
                  tunnel: w1064 -> [w1242]
                  tunnel: w1063 -> [w1243]
                  tunnel: [w1243] -> w1062
                  tunnel: [w1241] -> w1057
                  tunnel: w1056 -> [w1241]
                  tunnel: w1055 -> [w1240]
                  tunnel: [w1234] -> w1052
                  tunnel: w1051 -> [w1234]
                  tunnel: w1046 -> [w1232]
                  tunnel: [w1233] -> w1045
                  tunnel: w1044 -> [w1233]
                  tunnel: w1039 -> [w1230]
                  tunnel: [w1231] -> w1038
                  tunnel: w1037 -> [w1231]
                  tunnel: [w1229] -> w1032
                  tunnel: w1031 -> [w1229]
                  tunnel: w1030 -> [w1228]
                  tunnel: [w1217] -> w1024
                  tunnel: w1023 -> [w1217]
                  tunnel: [w1216] -> w1022
                  tunnel: w1021 -> [w1216]
                  tunnel: [w1214] -> w1010
                  tunnel: w1009 -> [w1214]
                  tunnel: [w1213] -> w1008
                  tunnel: w1007 -> [w1213]
                  tunnel: w1006 -> [w1211]
                  tunnel: w1005 -> [w1212]
                  tunnel: [w1210] -> w996
                  tunnel: w995 -> [w1210]
                  tunnel: [w1209] -> w994
                  tunnel: w993 -> [w1209]
                  tunnel: w992 -> [w1207]
                  tunnel: w991 -> [w1208]
                  tunnel: [w1206] -> w982
                  tunnel: w981 -> [w1206]
                  tunnel: [w1205] -> w980
                  tunnel: w979 -> [w1205]
                  tunnel: w978 -> [w1204]
                  tunnel: w977 -> [w1203]
                  tunnel: [w1202] -> w968
                  tunnel: w967 -> [w1202]
                  tunnel: [w1201] -> w966
                  tunnel: w965 -> [w1201]
                  tunnel: w964 -> [w1200]
                  tunnel: w963 -> [w1199]
                  tunnel: [w1188] -> w958
                  tunnel: w957 -> [w1188]
                  tunnel: [w1187] -> w956
                  tunnel: w955 -> [w1187]
                  tunnel: [w1186] -> w944
                  tunnel: w943 -> [w1186]
                  tunnel: [w1185] -> w942
                  tunnel: w941 -> [w1185]
                  tunnel: w940 -> [w1184]
                  tunnel: w939 -> [w1183]
                  tunnel: [w1182] -> w930
                  tunnel: w929 -> [w1182]
                  tunnel: [w1181] -> w928
                  tunnel: w927 -> [w1181]
                  tunnel: w926 -> [w1179]
                  tunnel: w925 -> [w1180]
                  tunnel: w1178 -> [w1429]
                  tunnel: w1177 -> [w1428]
                  tunnel: w1176 -> [w1427]
                  tunnel: w1175 -> [w1426]
                  tunnel: w1174 -> [w1425]
                  tunnel: w1173 -> [w1424]
                  tunnel: w1172 -> [w1423]
                  tunnel: w1171 -> [w1422]
                  tunnel: [w1391] -> w1170
                  tunnel: [w1392] -> w1169
                  tunnel: [w1386] -> w1168
                  tunnel: [w1385] -> w1167
                  tunnel: w1166 -> [w1409]
                  tunnel: [w1391] -> w1163
                  tunnel: [w1391] -> w1162
                  tunnel: [w1420] -> w1160
                  tunnel: [w1421] -> w1159
                  tunnel: w1157 -> [w1421]
                  tunnel: w1154 -> [w1420]
                  tunnel: [w1392] -> w1152
                  tunnel: [w1392] -> w1151
                  tunnel: [w1386] -> w1150
                  tunnel: [w1386] -> w1149
                  tunnel: [w1385] -> w1148
                  tunnel: [w1385] -> w1147
                  tunnel: w1142 -> [w1419]
                  tunnel: w1140 -> [w1418]
                  tunnel: [w1419] -> w1138
                  tunnel: [w1418] -> w1137
                  tunnel: w1119 -> [w1417]
                  tunnel: w1118 -> [w1416]
                  tunnel: w1117 -> [w1415]
                  tunnel: [w1417] -> w1116
                  tunnel: [w1416] -> w1115
                  tunnel: [w1415] -> w1114
                  tunnel: w1111 -> [w1414]
                  tunnel: [w1414] -> w1110
                  tunnel: [w1391] -> w1107
                  tunnel: [w1391] -> w1106
                  tunnel: w1105 -> [w1413]
                  tunnel: [w1413] -> w1103
                  tunnel: [w1392] -> w1102
                  tunnel: [w1386] -> w1101
                  tunnel: [w1385] -> w1100
                  tunnel: w1093 -> [w1412]
                  tunnel: w1091 -> [w1411]
                  tunnel: w1089 -> [w1410]
                  tunnel: [w1412] -> w1084
                  tunnel: [w1411] -> w1083
                  tunnel: [w1410] -> w1082
                  tunnel: [w1391] -> w1080
                  tunnel: [w1408] -> w1079
                  tunnel: w1077 -> [w1408]
                  tunnel: [w1392] -> w1073
                  tunnel: [w1407] -> w1072
                  tunnel: w1071 -> [w1407]
                  tunnel: [w1386] -> w1068
                  tunnel: [w1406] -> w1067
                  tunnel: w1062 -> [w1406]
                  tunnel: [w1385] -> w1061
                  tunnel: [w1405] -> w1060
                  tunnel: w1057 -> [w1405]
                  tunnel: [w1391] -> w1053
                  tunnel: w1052 -> [w1404]
                  tunnel: [w1404] -> w1050
                  tunnel: [w1392] -> w1049
                  tunnel: w1045 -> [w1403]
                  tunnel: [w1403] -> w1043
                  tunnel: [w1386] -> w1042
                  tunnel: w1038 -> [w1402]
                  tunnel: [w1402] -> w1036
                  tunnel: [w1385] -> w1035
                  tunnel: w1032 -> [w1401]
                  tunnel: [w1401] -> w1029
                  tunnel: [w1391] -> w1028
                  tunnel: [w1391] -> w1027
                  tunnel: w1024 -> [w1400]
                  tunnel: w1022 -> [w1399]
                  tunnel: [w1400] -> w1020
                  tunnel: [w1399] -> w1019
                  tunnel: [w1392] -> w1018
                  tunnel: [w1392] -> w1017
                  tunnel: [w1397] -> w1012
                  tunnel: [w1398] -> w1011
                  tunnel: w1010 -> [w1398]
                  tunnel: w1008 -> [w1397]
                  tunnel: [w1386] -> w1004
                  tunnel: [w1396] -> w1001
                  tunnel: [w1386] -> w1000
                  tunnel: [w1395] -> w997
                  tunnel: w996 -> [w1396]
                  tunnel: w994 -> [w1395]
                  tunnel: [w1385] -> w990
                  tunnel: [w1385] -> w989
                  tunnel: [w1394] -> w984
                  tunnel: [w1393] -> w983
                  tunnel: w982 -> [w1393]
                  tunnel: w980 -> [w1394]
                  tunnel: [w1392] -> w976
                  tunnel: [w1392] -> w975
                  tunnel: [w1388] -> w974
                  tunnel: [w1387] -> w973
                  tunnel: w968 -> [w1388]
                  tunnel: w966 -> [w1387]
                  tunnel: [w1391] -> w962
                  tunnel: [w1391] -> w961
                  tunnel: w958 -> [w1390]
                  tunnel: w956 -> [w1389]
                  tunnel: [w1390] -> w954
                  tunnel: [w1389] -> w953
                  tunnel: [w1386] -> w952
                  tunnel: [w1386] -> w951
                  tunnel: [w1384] -> w946
                  tunnel: [w1383] -> w945
                  tunnel: w944 -> [w1384]
                  tunnel: w942 -> [w1383]
                  tunnel: [w1385] -> w938
                  tunnel: [w1385] -> w937
                  tunnel: [w1382] -> w936
                  tunnel: [w1381] -> w935
                  tunnel: w930 -> [w1382]
                  tunnel: w928 -> [w1381]
                  tunnel: w1170 -> [_]
                  tunnel: w1169 -> [_]
                  tunnel: w1168 -> [_]
                  tunnel: w1167 -> [_]
                  tunnel: w1163 -> [w1632]
                  tunnel: w1162 -> [w1631]
                  tunnel: w1161 -> [w1460]
                  tunnel: w1160 -> [w1630]
                  tunnel: w1159 -> [w1629]
                  tunnel: [w1579] -> w1158
                  tunnel: [w1578] -> w1155
                  tunnel: w1152 -> [w1616]
                  tunnel: w1151 -> [w1615]
                  tunnel: w1150 -> [w1614]
                  tunnel: w1149 -> [w1613]
                  tunnel: w1148 -> [w1612]
                  tunnel: w1147 -> [w1611]
                  tunnel: [w1610] -> w1146
                  tunnel: [w1610] -> w1145
                  tunnel: [w1609] -> w1144
                  tunnel: [w1609] -> w1143
                  tunnel: w1138 -> [w1608]
                  tunnel: w1137 -> [w1607]
                  tunnel: [w1606] -> w1134
                  tunnel: [w1606] -> w1133
                  tunnel: [w1605] -> w1132
                  tunnel: [w1605] -> w1131
                  tunnel: [w1604] -> w1130
                  tunnel: [w1603] -> w1129
                  tunnel: [w1604] -> w1128
                  tunnel: [w1603] -> w1127
                  tunnel: w1116 -> [w1602]
                  tunnel: w1115 -> [w1601]
                  tunnel: w1114 -> [w1600]
                  tunnel: w1110 -> [w1599]
                  tunnel: [w1577] -> w1108
                  tunnel: w1107 -> [w1596]
                  tunnel: w1106 -> [_]
                  tunnel: w1103 -> [w1595]
                  tunnel: w1102 -> [w1588]
                  tunnel: w1101 -> [w1587]
                  tunnel: w1100 -> [w1586]
                  tunnel: [w1585] -> w1099
                  tunnel: [w1584] -> w1098
                  tunnel: [w1583] -> w1097
                  tunnel: [w1585] -> w1096
                  tunnel: [w1584] -> w1095
                  tunnel: [w1583] -> w1094
                  tunnel: w1084 -> [w1582]
                  tunnel: w1083 -> [w1581]
                  tunnel: w1082 -> [w1580]
                  tunnel: w1080 -> [w1574]
                  tunnel: [w1573] -> w1078
                  tunnel: w1079 -> [w1572]
                  tunnel: [w1569] -> w1074
                  tunnel: [w1569] -> w1075
                  tunnel: w1073 -> [w1568]
                  tunnel: w1072 -> [w1567]
                  tunnel: w1068 -> [w1564]
                  tunnel: w1067 -> [w1563]
                  tunnel: [w1562] -> w1066
                  tunnel: [w1562] -> w1065
                  tunnel: w1061 -> [w1559]
                  tunnel: w1060 -> [w1558]
                  tunnel: [w1557] -> w1059
                  tunnel: [w1557] -> w1058
                  tunnel: [w1554] -> w1054
                  tunnel: w1053 -> [w1553]
                  tunnel: w1050 -> [w1552]
                  tunnel: w1049 -> [w1549]
                  tunnel: [w1548] -> w1047
                  tunnel: [w1548] -> w1048
                  tunnel: w1043 -> [w1547]
                  tunnel: [w1544] -> w1041
                  tunnel: [w1544] -> w1040
                  tunnel: w1042 -> [w1543]
                  tunnel: w1036 -> [w1542]
                  tunnel: w1035 -> [w1539]
                  tunnel: [w1538] -> w1034
                  tunnel: [w1538] -> w1033
                  tunnel: w1029 -> [w1537]
                  tunnel: w1028 -> [w1532]
                  tunnel: w1027 -> [w1531]
                  tunnel: [w1530] -> w1026
                  tunnel: [w1529] -> w1025
                  tunnel: w1020 -> [w1528]
                  tunnel: w1019 -> [w1527]
                  tunnel: w1018 -> [w1522]
                  tunnel: w1017 -> [w1521]
                  tunnel: [w1520] -> w1016
                  tunnel: [w1520] -> w1015
                  tunnel: [w1519] -> w1014
                  tunnel: [w1519] -> w1013
                  tunnel: w1012 -> [w1518]
                  tunnel: w1011 -> [w1517]
                  tunnel: w1004 -> [w1514]
                  tunnel: [w1513] -> w1003
                  tunnel: [w1513] -> w1002
                  tunnel: w1001 -> [w1512]
                  tunnel: w1000 -> [w1509]
                  tunnel: [w1508] -> w999
                  tunnel: [w1508] -> w998
                  tunnel: w997 -> [w1507]
                  tunnel: w990 -> [w1502]
                  tunnel: w989 -> [w1501]
                  tunnel: [w1500] -> w988
                  tunnel: [w1500] -> w987
                  tunnel: [w1499] -> w986
                  tunnel: [w1499] -> w985
                  tunnel: w984 -> [w1498]
                  tunnel: w983 -> [w1497]
                  tunnel: w976 -> [w1492]
                  tunnel: w975 -> [w1491]
                  tunnel: w974 -> [w1490]
                  tunnel: w973 -> [w1489]
                  tunnel: [w1488] -> w972
                  tunnel: [w1488] -> w970
                  tunnel: [w1487] -> w971
                  tunnel: [w1487] -> w969
                  tunnel: w962 -> [w1482]
                  tunnel: w961 -> [w1481]
                  tunnel: [w1480] -> w960
                  tunnel: [w1479] -> w959
                  tunnel: w954 -> [w1478]
                  tunnel: w953 -> [w1477]
                  tunnel: w952 -> [w1472]
                  tunnel: w951 -> [w1471]
                  tunnel: [w1470] -> w950
                  tunnel: [w1470] -> w948
                  tunnel: [w1469] -> w949
                  tunnel: [w1469] -> w947
                  tunnel: w946 -> [w1468]
                  tunnel: w945 -> [w1467]
                  tunnel: w938 -> [w1462]
                  tunnel: w937 -> [w1461]
                  tunnel: w936 -> [w1459]
                  tunnel: w935 -> [w1458]
                  tunnel: [w1457] -> w932
                  tunnel: [w1457] -> w934
                  tunnel: [w1456] -> w931
                  tunnel: [w1456] -> w933
                  frame #0 {
                    n291 = case shown="1, Default" w1299 {
                      tunnel: [w1308 w1317 w1321 w1335 w1340 w1348 w1358 w1363 w1376] -> w1295
                      tunnel: [w1307 w1313 w1322 w1331 w1341 w1349 w1354 w1364 w1377] -> w1294
                      tunnel: [w1306 w1314 w1323 w1332 w1342 w1350 w1355 w1365 w1378] -> w1293
                      tunnel: [w1304 w1315 w1324 w1333 w1343 w1351 w1356 w1366 w1379] -> w1292
                      tunnel: [w1305 w1316 w1325 w1334 w1344 w1352 w1357 w1367 w1380] -> w1291
                      tunnel: "sos gain SF Controller xx1" -> [w1308 _ _ _ _ _ _ _ _]
                      tunnel: "-a01(2) xx1" -> [w1307 _ _ _ _ _ _ _ _]
                      tunnel: "-a02(2) xx1" -> [w1306 _ _ _ _ _ _ _ _]
                      tunnel: "b01(2) xx1" -> [w1304 _ _ _ _ _ _ _ _]
                      tunnel: "b02(2) xx1" -> [w1305 _ _ _ _ _ _ _ _]
                      tunnel: "sos gain SF Controller yy1" -> [_ _ _ _ w1340 _ _ _ _]
                      tunnel: "-a01(2) yy1" -> [_ _ _ _ w1341 _ _ _ _]
                      tunnel: "-a02(2) yy1" -> [_ _ _ _ w1342 _ _ _ _]
                      tunnel: "b01(2) yy1" -> [_ _ _ _ w1343 _ _ _ _]
                      tunnel: "b02(2) yy1" -> [_ _ _ _ w1344 _ _ _ _]
                      tunnel: [w1301 w1310 w1320 w1329 w1339 w1347 w1362 w1371 w1375] -> w1296
                      tunnel: [w1302 w1311 w1319 w1328 w1338 w1346 w1361 w1370 w1374] -> w1297
                      tunnel: [w1303 w1312 w1318 w1327 w1337 w1345 w1360 w1369 w1373] -> w1298
                      tunnel: w1279 -> [w1303 _ _ _ _ _ _ _ _]
                      tunnel: w1280 -> [_ _ _ _ w1337 _ _ _ _]
                      tunnel: w1281 -> [w1302 _ _ _ _ _ _ _ _]
                      tunnel: w1282 -> [_ _ _ _ w1338 _ _ _ _]
                      tunnel: w1283 -> [w1301 _ _ _ _ _ _ _ _]
                      tunnel: w1284 -> [_ _ _ _ w1339 _ _ _ _]
                      tunnel: [w1300 w1309 w1326 w1330 w1336 w1353 w1359 w1368 w1372] -> w1277
                      tunnel: w1253 -> [w1300 _ _ w1330 _ _ w1359 _ _]
                      tunnel: "sos gain SF Controller zz1" -> [_ _ _ _ _ _ _ _ w1376]
                      tunnel: "-a01(2) zz1" -> [_ _ _ _ _ _ _ _ w1377]
                      tunnel: "-a02(2) zz1" -> [_ _ _ _ _ _ _ _ w1378]
                      tunnel: "b01(2) zz1" -> [_ _ _ _ _ _ _ _ w1379]
                      tunnel: "b02(2) zz1" -> [_ _ _ _ _ _ _ _ w1380]
                      tunnel: w1275 -> [_ w1309 _ _ w1336 _ _ w1368 _]
                      tunnel: w1271 -> [_ _ _ _ _ _ _ _ w1375]
                      tunnel: w1270 -> [_ _ _ _ _ _ _ _ w1374]
                      tunnel: w1269 -> [_ _ _ _ _ _ _ _ w1373]
                      tunnel: w1252 -> [_ _ w1326 _ _ w1353 _ _ w1372]
                      tunnel: "sos gain SF Controller yx1" -> [_ w1317 _ _ _ _ _ _ _]
                      tunnel: "-a01(2) yx1" -> [_ w1313 _ _ _ _ _ _ _]
                      tunnel: "-a02(2) yx1" -> [_ w1314 _ _ _ _ _ _ _]
                      tunnel: "b01(2) yx1" -> [_ w1315 _ _ _ _ _ _ _]
                      tunnel: "b02(2) yx1" -> [_ w1316 _ _ _ _ _ _ _]
                      tunnel: w1244 -> [_ w1312 _ _ _ _ _ _ _]
                      tunnel: w1242 -> [_ w1311 _ _ _ _ _ _ _]
                      tunnel: w1240 -> [_ w1310 _ _ _ _ _ _ _]
                      tunnel: "sos gain SF Controller zx1" -> [_ _ w1321 _ _ _ _ _ _]
                      tunnel: "-a01(2) zx1" -> [_ _ w1322 _ _ _ _ _ _]
                      tunnel: "-a02(2) zx1" -> [_ _ w1323 _ _ _ _ _ _]
                      tunnel: "b01(2) zx1" -> [_ _ w1324 _ _ _ _ _ _]
                      tunnel: "b02(2) zx1" -> [_ _ w1325 _ _ _ _ _ _]
                      tunnel: w1228 -> [_ _ w1320 _ _ _ _ _ _]
                      tunnel: w1230 -> [_ _ w1319 _ _ _ _ _ _]
                      tunnel: w1232 -> [_ _ w1318 _ _ _ _ _ _]
                      tunnel: "sos gain SF Controller xy1" -> [_ _ _ w1335 _ _ _ _ _]
                      tunnel: "-a01(2) xy1" -> [_ _ _ w1331 _ _ _ _ _]
                      tunnel: "-a02(2) xy1" -> [_ _ _ w1332 _ _ _ _ _]
                      tunnel: "b01(2) xy1" -> [_ _ _ w1333 _ _ _ _ _]
                      tunnel: "b02(2) xy1" -> [_ _ _ w1334 _ _ _ _ _]
                      tunnel: "sos gain SF Controller zy1" -> [_ _ _ _ _ w1348 _ _ _]
                      tunnel: "-a01(2) zy1" -> [_ _ _ _ _ w1349 _ _ _]
                      tunnel: "-a02(2) zy1" -> [_ _ _ _ _ w1350 _ _ _]
                      tunnel: "b01(2) zy1" -> [_ _ _ _ _ w1351 _ _ _]
                      tunnel: "b02(2) zy1" -> [_ _ _ _ _ w1352 _ _ _]
                      tunnel: w1203 -> [_ _ _ _ _ w1347 _ _ _]
                      tunnel: w1208 -> [_ _ _ _ _ w1346 _ _ _]
                      tunnel: w1212 -> [_ _ _ _ _ w1345 _ _ _]
                      tunnel: w1204 -> [_ _ _ w1329 _ _ _ _ _]
                      tunnel: w1207 -> [_ _ _ w1328 _ _ _ _ _]
                      tunnel: w1211 -> [_ _ _ w1327 _ _ _ _ _]
                      tunnel: w1180 -> [_ _ _ _ _ _ _ w1371 _]
                      tunnel: w1179 -> [_ _ _ _ _ _ w1362 _ _]
                      tunnel: w1183 -> [_ _ _ _ _ _ _ w1370 _]
                      tunnel: w1184 -> [_ _ _ _ _ _ w1361 _ _]
                      tunnel: w1199 -> [_ _ _ _ _ _ _ w1369 _]
                      tunnel: w1200 -> [_ _ _ _ _ _ w1360 _ _]
                      tunnel: "sos gain SF Controller xz1" -> [_ _ _ _ _ _ w1358 _ _]
                      tunnel: "-a01(2) xz1" -> [_ _ _ _ _ _ w1354 _ _]
                      tunnel: "-a02(2) xz1" -> [_ _ _ _ _ _ w1355 _ _]
                      tunnel: "b01(2) xz1" -> [_ _ _ _ _ _ w1356 _ _]
                      tunnel: "b02(2) xz1" -> [_ _ _ _ _ _ w1357 _ _]
                      tunnel: "sos gain SF Controller yz1" -> [_ _ _ _ _ _ _ w1363 _]
                      tunnel: "-a01(2) yz1" -> [_ _ _ _ _ _ _ w1364 _]
                      tunnel: "-a02(2) yz1" -> [_ _ _ _ _ _ _ w1365 _]
                      tunnel: "b01(2) yz1" -> [_ _ _ _ _ _ _ w1366 _]
                      tunnel: "b02(2) yz1" -> [_ _ _ _ _ _ _ w1367 _]
                      frame 1, Default {
                      }
                      frame 2 {
                      }
                      frame 3 {
                      }
                      frame 4 {
                      }
                      frame 5 {
                      }
                      frame 6 {
                      }
                      frame 7 {
                      }
                      frame 8 {
                      }
                      frame 9 {
                      }
                    }
                  }
                  frame #1 {
                    n292 = Multiply(x=w1409, y=w1426) -> (x*y=w1430:fxp<+/-,64,34>)
                    n293 = To Fixed-Point(number=w1430) -> (fixed-point=w1431:fxp<+/-,58,25>)  [unwired: 1 in]
                    n294 = for {
                      tunnel: w1425 -> [w1447] mode=indexing
                      tunnel: w1422 -> [w1444] mode=indexing
                      shift-right: [w1449] -> w1391
                      shift-left: w1431 -> [w1448]
                      tunnel: w1424 -> [w1446] mode=indexing
                      tunnel: w1423 -> [w1445] mode=indexing
                      tunnel: [w1436] -> w1392 mode=indexing
                      tunnel: w1429 -> [w1442] mode=indexing
                      tunnel: [w1439] -> w1386 mode=indexing
                      tunnel: w1428 -> [w1432] mode=indexing
                      tunnel: [w1432] -> w1385 mode=indexing
                      tunnel: w1427 -> [w1440] mode=indexing
                      n295 = To Fixed-Point(number=w1442) -> (fixed-point=w1455:fxp<+/-,58,25>)  [unwired: 1 in]
                      n296 = Add(x=w1448, y=w1455) -> (x+y=w1441:fxp<+/-,59,26>)
                      n297 = To Fixed-Point(number=w1441) -> (fixed-point=w1439:fxp<+/-,58,25>)  [unwired: 1 in]
                      n298 = Multiply(x=w1439, y=w1447) -> (x*y=w1454:fxp<+/-,64,34>)
                      n299 = To Fixed-Point(number=w1454) -> (fixed-point=w1435:fxp<+/-,58,25>)  [unwired: 1 in]
                      n300 = Multiply(x=w1432, y=w1446) -> (x*y=w1450:fxp<+/-,64,34>)
                      n301 = To Fixed-Point(number=w1450) -> (fixed-point=w1434:fxp<+/-,58,25>)  [unwired: 1 in]
                      n302 = Add(x=w1435, y=w1434) -> (x+y=w1443:fxp<+/-,59,26>)
                      n303 = To Fixed-Point(number=w1443) -> (fixed-point=w1436:fxp<+/-,58,25>)  [unwired: 1 in]
                      n304 = Multiply(x=w1432, y=w1445) -> (x*y=w1451:fxp<+/-,64,34>)
                      n305 = Multiply(x=w1440, y=w1444) -> (x*y=w1453:fxp<+/-,64,34>)
                      n306 = To Fixed-Point(number=w1451) -> (fixed-point=w1437:fxp<+/-,58,25>)  [unwired: 1 in]
                      n307 = To Fixed-Point(number=w1453) -> (fixed-point=w1433:fxp<+/-,58,25>)  [unwired: 1 in]
                      n308 = Add(x=w1437, y=w1433) -> (x+y=w1452:fxp<+/-,59,26>)
                      n309 = To Fixed-Point(number=w1452) -> (fixed-point=w1438:fxp<+/-,58,25>)  [unwired: 1 in]
                      n310 = Add(x=w1439, y=w1438) -> (x+y=w1449:fxp<+/-,58,25>)
                    }
                  }
                  frame #2 {
                    n311 = Equal?(x=6, y=w1460) -> (x = y?=w1533:bool)
                    n312 = Equal?(x=5, y=w1460) -> (x = y?=w1633:bool)
                    n313 = Equal?(x=1, y=w1460) -> (x = y?=w1635:bool)
                    n314 = Equal?(x=9, y=w1460) -> (x = y?=w1597:bool)
                    n315 = Equal?(x=2, y=w1460) -> (x = y?=w1575:bool)
                    n316 = Equal?(x=4, y=w1460) -> (x = y?=w1535:bool)
                    n317 = Equal?(x=7, y=w1460) -> (x = y?=w1483:bool)
                    n318 = Equal?(x=3, y=w1460) -> (x = y?=w1555:bool)
                    n319 = Equal?(x=8, y=w1460) -> (x = y?=w1485:bool)
                    n320 = Equal?(x=6, y=w1460) -> (x = y?=w1503:bool)
                    n321 = Equal?(x=5, y=w1460) -> (x = y?=w1625:bool)
                    n322 = Equal?(x=9, y=w1460) -> (x = y?=w1593:bool)
                    n323 = Equal?(x=5, y=w1460) -> (x = y?=w1621:bool)
                    n324 = Equal?(x=6, y=w1460) -> (x = y?=w1510:bool)
                    n325 = Equal?(x=4, y=w1460) -> (x = y?=w1505:bool)
                    n326 = Equal?(x=5, y=w1460) -> (x = y?=w1617:bool)
                    n327 = Equal?(x=7, y=w1460) -> (x = y?=w1465:bool)
                    n328 = Equal?(x=9, y=w1460) -> (x = y?=w1589:bool)
                    n329 = Equal?(x=1, y=w1460) -> (x = y?=w1627:bool)
                    n330 = Equal?(x=6, y=w1460) -> (x = y?=w1523:bool)
                    n331 = Equal?(x=1, y=w1460) -> (x = y?=w1623:bool)
                    n332 = Equal?(x=2, y=w1460) -> (x = y?=w1565:bool)
                    n333 = Equal?(x=4, y=w1460) -> (x = y?=w1515:bool)
                    n334 = Equal?(x=9, y=w1460) -> (x = y?=w1591:bool)
                    n335 = Equal?(x=1, y=w1460) -> (x = y?=w1619:bool)
                    n336 = Equal?(x=2, y=w1460) -> (x = y?=w1570:bool)
                    n337 = Equal?(x=7, y=w1460) -> (x = y?=w1495:bool)
                    n338 = Equal?(x=8, y=w1460) -> (x = y?=w1493:bool)
                    n339 = Equal?(x=2, y=w1460) -> (x = y?=w1560:bool)
                    n340 = Equal?(x=8, y=w1460) -> (x = y?=w1463:bool)
                    n341 = Equal?(x=4, y=w1460) -> (x = y?=w1525:bool)
                    n342 = Equal?(x=3, y=w1460) -> (x = y?=w1545:bool)
                    n343 = Equal?(x=3, y=w1460) -> (x = y?=w1540:bool)
                    n344 = Equal?(x=7, y=w1460) -> (x = y?=w1475:bool)
                    n345 = Equal?(x=8, y=w1460) -> (x = y?=w1473:bool)
                    n346 = Equal?(x=3, y=w1460) -> (x = y?=w1550:bool)
                    n347 = Select(t=w1531, s=w1533, f=w1527) -> (s? t:f=w1529:fxp<+/-,58,25>)
                    "Kzy Output, Kzy*ez (V)" <- w1529
                    n348 = Select(t=w1631, s=w1633, f=w1630) -> (s? t:f=w1578:fxp<+/-,58,25>)
                    "Kyy Output, Kyy*ey (V)" <- w1578
                    n349 = Select(t=w1632, s=w1635, f=w1629) -> (s? t:f=w1579:fxp<+/-,58,25>)
                    "Kxx Output, Kxx*ex (V)" <- w1579
                    n350 = Select(t=w1596, s=w1597, f=w1595) -> (s? t:f=w1577:fxp<+/-,58,25>)
                    "Kzz Output, Kzz*ez (V)" <- w1577
                    n351 = Select(t=w1532, s=w1535, f=w1528) -> (s? t:f=w1530:fxp<+/-,58,25>)
                    "Kxy Output, Kxy*ex (V)" <- w1530
                    n352 = Select(t=w1482, s=w1483, f=w1478) -> (s? t:f=w1480:fxp<+/-,58,25>)
                    "Kxz Output, Kxz*ex (V)" <- w1480
                    n353 = Select(t=w1574, s=w1575, f=w1572) -> (s? t:f=w1573:fxp<+/-,58,25>)
                    "Kyx Output, Kyx*ey (V)" <- w1573
                    n354 = Select(t=w1481, s=w1485, f=w1477) -> (s? t:f=w1479:fxp<+/-,58,25>)
                    "Kyz Output, Kyz*ey (V)" <- w1479
                    n355 = Select(t=w1553, s=w1555, f=w1552) -> (s? t:f=w1554:fxp<+/-,58,25>)
                    "Kzx Output, Kzx*ez (V)" <- w1554
                    n356 = Select(t=w1501, s=w1503, f=w1497) -> (s? t:f=w1499:fxp<+/-,58,25>[])
                    n357 = Select(t=w1615, s=w1625, f=w1607) -> (s? t:f=w1609:fxp<+/-,58,25>[])
                    n358 = Select(t=w1588, s=w1593, f=w1582) -> (s? t:f=w1585:fxp<+/-,58,25>[])
                    n359 = Select(t=w1613, s=w1621, f=w1601) -> (s? t:f=w1605:fxp<+/-,58,25>[])
                    n360 = Select(t=w1509, s=w1510, f=w1507) -> (s? t:f=w1508:fxp<+/-,58,25>[])
                    n361 = Select(t=w1502, s=w1505, f=w1498) -> (s? t:f=w1500:fxp<+/-,58,25>[])
                    n362 = Select(t=w1611, s=w1617, f=w1599) -> (s? t:f=w1603:fxp<+/-,58,25>[])
                    n363 = Select(t=w1462, s=w1465, f=w1459) -> (s? t:f=w1457:fxp<+/-,58,25>[])
                    n364 = Select(t=w1586, s=w1589, f=w1580) -> (s? t:f=w1583:fxp<+/-,58,25>[])
                    n365 = Select(t=w1616, s=w1627, f=w1608) -> (s? t:f=w1610:fxp<+/-,58,25>[])
                    n366 = Select(t=w1521, s=w1523, f=w1518) -> (s? t:f=w1519:fxp<+/-,58,25>[])
                    n367 = Select(t=w1614, s=w1623, f=w1602) -> (s? t:f=w1606:fxp<+/-,58,25>[])
                    n368 = Select(t=w1564, s=w1565, f=w1563) -> (s? t:f=w1562:fxp<+/-,58,25>[])
                    n369 = Select(t=w1514, s=w1515, f=w1512) -> (s? t:f=w1513:fxp<+/-,58,25>[])
                    n370 = Select(t=w1587, s=w1591, f=w1581) -> (s? t:f=w1584:fxp<+/-,58,25>[])
                    n371 = Select(t=w1612, s=w1619, f=w1600) -> (s? t:f=w1604:fxp<+/-,58,25>[])
                    n372 = Select(t=w1568, s=w1570, f=w1567) -> (s? t:f=w1569:fxp<+/-,58,25>[])
                    n373 = Select(t=w1492, s=w1495, f=w1490) -> (s? t:f=w1488:fxp<+/-,58,25>[])
                    n374 = Select(t=w1491, s=w1493, f=w1489) -> (s? t:f=w1487:fxp<+/-,58,25>[])
                    n375 = Select(t=w1559, s=w1560, f=w1558) -> (s? t:f=w1557:fxp<+/-,58,25>[])
                    n376 = Select(t=w1461, s=w1463, f=w1458) -> (s? t:f=w1456:fxp<+/-,58,25>[])
                    n377 = Select(t=w1522, s=w1525, f=w1517) -> (s? t:f=w1520:fxp<+/-,58,25>[])
                    n378 = Select(t=w1543, s=w1545, f=w1542) -> (s? t:f=w1544:fxp<+/-,58,25>[])
                    n379 = Select(t=w1539, s=w1540, f=w1537) -> (s? t:f=w1538:fxp<+/-,58,25>[])
                    n380 = Select(t=w1472, s=w1475, f=w1468) -> (s? t:f=w1470:fxp<+/-,58,25>[])
                    n381 = Select(t=w1471, s=w1473, f=w1467) -> (s? t:f=w1469:fxp<+/-,58,25>[])
                    n382 = Select(t=w1549, s=w1550, f=w1547) -> (s? t:f=w1548:fxp<+/-,58,25>[])
                  }
                }
              }
              n383 = Add(x=w866, y=w867) -> (x+y=w868:fxp<+/-,59,26>)
              n384 = Add(x=w845, y=w846) -> (x+y=w847:fxp<+/-,59,26>)
              n385 = Add(x=w878, y=w879) -> (x+y=w877:fxp<+/-,59,26>)
              n386 = Add(x=w865, y=w868) -> (x+y=w864:fxp<+/-,60,27>)
              n387 = Add(x=w844, y=w847) -> (x+y=w843:fxp<+/-,60,27>)
              n388 = Add(x=w876, y=w877) -> (x+y=w875:fxp<+/-,60,27>)
              n389 = Multiply(x=w843, y="Scaling mV to V") -> (x*y=w916:fxp<+/-,64,37>)
              n390 = Multiply(x=w875, y="Scaling mV to V") -> (x*y=w915:fxp<+/-,64,37>)
              n391 = Multiply(x=w864, y="Scaling mV to V") -> (x*y=w894:fxp<+/-,64,37>)
              n392 = To Fixed-Point(fixed-point type=w886, number=w915) -> (fixed-point=w917:fxp<+/-,58,25>)
              n393 = To Fixed-Point(fixed-point type=w886, number=w894) -> (fixed-point=w892:fxp<+/-,58,25>)
              n394 = To Fixed-Point(fixed-point type=w886, number=w916) -> (fixed-point=w893:fxp<+/-,58,25>)
            }
          }
          n395 = To Fixed-Point(fixed-point type=w760, number=w764) -> (fixed-point=w763:fxp<+/-,20,5>)
          n396 = To Fixed-Point(fixed-point type=w760, number=w784) -> (fixed-point=w762:fxp<+/-,20,5>)
          n397 = To Fixed-Point(fixed-point type=w760, number=w783) -> (fixed-point=w761:fxp<+/-,20,5>)
          n398 = call "measure_loop_rate_FPGA.vi"() -> ("Loop Rate (Ticks)"=→"Measured Controller Time Period (Ticks)":u32)  [unwired: 11 in]
          n399 = In Range and Coerce(upper limit="Controller Output Upper Limit", x=w763, lower limit="Controller Output Lower Limit") -> (coerced(x)=→"PI X-Stage Input (V)":fxp<+/-,20,5>, In Range?=→"X-Stage Input In Range?":bool)
          n400 = In Range and Coerce(upper limit="Controller Output Upper Limit", x=w762, lower limit="Controller Output Lower Limit") -> (coerced(x)=→"PI Y-Stage Input (V)":fxp<+/-,20,5>, In Range?=→"Y-Stage Input In Range?":bool)
          n401 = In Range and Coerce(upper limit="Controller Output Upper Limit", x=w761, lower limit="Controller Output Lower Limit") -> (coerced(x)=→"PI Z-Stage Input (V)":fxp<+/-,20,5>, In Range?=→"Z-Stage Input In Range?":bool)
          n402 = local read "stop case"() -> (w795:bool)
        }
        n403 = while {
          tunnel: [w1653] -> w114
          shift-right: [w1646] -> _
          shift-left: _ -> [w1645]
          shift-right: [w1642] -> _
          shift-left: _ -> [w1641]
          stop <- w1651 stop-if-true
          n404 = local read "Detector Trigger (V)"() -> (w1646:fxp<+/-,20,5>)
          n405 = local read "Trigger for Data"() -> (w1642:fxp<+/-,58,25>)
          n406 = local read "Fly Scan Running"() -> (w1643:bool)
          n407 = Greater?(x=w1646, y=w1645) -> (0:w1644:bool)
          n408 = Greater?(x=w1642, y=w1641) -> (0:w1640:bool)
          n409 = case shown="True" w1643 {
            tunnel: [w1657 w1670] -> w1654
            tunnel: [w1658 w1669] -> w1647
            tunnel: w1644 -> [_ w1668]
            tunnel: w1640 -> [w1656 _]
            frame False {
              w1665 = 5  # # of Data Strings
              n410 = case shown="True" w1656 {
                tunnel: w1665 -> [_ w1666]
                tunnel: fxp<+/-,58,25> 0.0 ("fixed-point type") -> [_ w1667]
                tunnel: [_ w1667] -> w1663
                tunnel: [_ w1667] -> w1661
                tunnel: [_ w1667] -> w1660
                tunnel: [_ w1667] -> w1659
                tunnel: [_ w1667] -> w1662
                tunnel: [_ w1666] -> w1657
                frame False {
                }
                frame True {
                }
              }
              "Number of Data Strings 2" <- w1657
              n411 = Build Array "Build Array"(w1663, w1662, w1661, w1660, w1659) -> (w1658:fxp<+/-,58,25>[])
            }
            frame True {
              n412 = case shown="True" w1668 {
                tunnel: [_ w1677] -> w1670
                tunnel: [_ w1673] -> w1669
                frame False {
                }
                frame True {
                  w1678 = 5  # # of Data Strings
                  n413 = local read "Sample X Stage Displacement (nm)"() -> (w1684:fxp<+/-,58,25>)
                  n414 = local read "Sample Y Stage Displacement (nm)"() -> (w1683:fxp<+/-,58,25>)
                  n415 = local read "Sample Z Stage Displacement (nm)"() -> (w1682:fxp<+/-,58,25>)
                  n416 = local read "Optics X Stage Displacement (nm)"() -> (w1688:fxp<+/-,58,25>)
                  n417 = local read "Optics Y Stage Displacement (nm)"() -> (w1687:fxp<+/-,58,25>)
                  n418 = local read "Optics Z Stage Displacement (nm)"() -> (w1685:fxp<+/-,58,25>)
                  n419 = local read "X Stage External Reference (nm)"() -> (w1676:fxp<+/-,58,25>)
                  n420 = local read "Y Stage External Reference (nm)"() -> (w1675:fxp<+/-,58,25>)
                  n421 = local read "Z Stage External Reference (nm)"() -> (w1674:fxp<+/-,58,25>)
                  n422 = local read "X Stage Reference (nm)"() -> (w1696:fxp<+/-,58,25>)
                  n423 = local read "Y Stage Reference (nm)"() -> (w1681:fxp<+/-,58,25>)
                  n424 = local read "Z Stage Reference (nm)"() -> (w1680:fxp<+/-,58,25>)
                  n425 = local read "Detector Trigger (V)"() -> (w1672:fxp<+/-,20,5>)
                  n426 = local read "PI X-Stage Input (V)"() -> (w1695:fxp<+/-,20,5>)
                  n427 = local read "PI Y-Stage Input (V)"() -> (w1694:fxp<+/-,20,5>)
                  n428 = local read "PI Z-Stage Input (V)"() -> (w1693:fxp<+/-,20,5>)
                  n429 = case shown="\"Data Log 16\"" "Datalog Cases" {
                    tunnel: fxp<+/-,58,25> 0.0 ("fixed-point type") -> [w1698 w1711 w1720 w1733 w1742 w1757 w1770 w1782 w1800 w1812 w1822 w1834 w1845 w1857 w1868 w1880]
                    tunnel: [w1707 w1718 w1730 w1741 w1754 w1767 w1777 w1794 w1804 w1818 w1827 w1842 w1854 w1865 w1876 w1888] -> w1691
                    tunnel: w1696 -> [w1708 _ _ _ w1747 _ _ _ _ _ _ _ _ _ _ w1884]
                    tunnel: w1695 -> [w1704 _ _ _ w1746 _ _ _ _ w1819 _ _ w1849 _ _ _]
                    tunnel: w1694 -> [_ w1717 _ _ _ w1761 _ _ _ _ w1832 _ _ w1860 _ _]
                    tunnel: w1693 -> [_ _ w1727 _ _ _ w1774 _ _ _ _ w1843 _ _ w1871 _]
                    tunnel: [w1706 w1710 w1729 w1735 w1753 w1766 w1776 w1790 w1803 w1813 w1826 w1841 w1853 w1864 w1875 w1887] -> w1690
                    tunnel: [w1705 w1719 w1728 w1740 w1752 w1765 w1775 w1786 w1802 w1814 w1825 w1840 w1852 w1863 w1874 w1886] -> w1689
                    tunnel: w1688 -> [w1701 _ _ w1737 w1749 _ _ w1797 _ w1817 w1831 w1838 w1848 _ _ w1882]
                    tunnel: w1687 -> [_ w1713 _ w1736 _ w1760 _ w1793 _ w1816 w1830 w1837 _ w1859 _ w1881]
                    tunnel: fxp<+/-,40,17> 0.0 ("fixed-point type") -> [w1700 w1712 w1722 w1731 w1744 w1756 w1768 w1781 w1798 w1809 w1821 w1833 w1847 w1856 w1867 _]
                    tunnel: w1685 -> [_ _ w1723 w1734 _ _ w1773 w1789 _ w1810 w1829 w1836 _ _ w1870 _]
                    tunnel: w1684 -> [_ _ _ _ w1748 _ _ w1796 w1807 _ _ _ _ _ _ _]
                    tunnel: w1683 -> [_ _ _ _ _ w1759 _ w1792 w1806 _ _ _ _ _ _ _]
                    tunnel: w1682 -> [_ _ _ _ _ _ w1772 w1788 w1805 _ _ _ _ _ _ _]
                    tunnel: w1681 -> [_ w1716 _ _ _ w1762 _ _ _ _ _ _ _ _ _ w1883]
                    tunnel: w1680 -> [_ _ w1726 _ _ _ w1778 _ _ _ _ _ _ _ _ _]
                    tunnel: [w1703 w1715 w1725 w1739 w1751 w1764 w1771 w1785 w1801 w1815 w1824 w1839 w1851 w1862 w1873 w1885] -> w1679
                    tunnel: w1678 -> [w1702 w1714 w1724 w1738 w1750 w1763 w1779 w1784 w1808 w1820 w1828 w1844 w1855 w1866 w1877 w1889]
                    tunnel: [w1702 w1714 w1724 w1738 w1750 w1763 w1779 w1784 w1808 w1820 w1828 w1844 w1855 w1866 w1877 w1889] -> w1677
                    tunnel: w1676 -> [_ _ _ _ _ _ _ _ _ _ _ _ w1850 _ _ _]
                    tunnel: w1675 -> [_ _ _ _ _ _ _ _ _ _ _ _ _ w1861 _ _]
                    tunnel: w1674 -> [_ _ _ _ _ _ _ _ _ _ _ _ _ _ w1872 _]
                    tunnel: w1672 -> [_ _ _ _ _ _ _ _ _ _ _ _ _ _ _ w1879]
                    tunnel: [w1699 w1709 w1721 w1732 w1743 w1755 w1769 w1783 w1799 w1811 w1823 w1835 w1846 w1858 w1869 w1878] -> w1671
                    frame "Data Log 1", Default {
                      n430 = To Fixed-Point(fixed-point type=w1698, number=w1708) -> (fixed-point=w1707:fxp<+/-,58,25>)
                      n431 = To Fixed-Point(fixed-point type=w1698, number=w1704) -> (fixed-point=w1706:fxp<+/-,58,25>)
                      n432 = To Fixed-Point(fixed-point type=w1698, number=w1701) -> (fixed-point=w1705:fxp<+/-,58,25>)
                      n433 = To Fixed-Point(fixed-point type=w1698, number=w1700) -> (fixed-point=w1703:fxp<+/-,58,25>)
                      n434 = To Fixed-Point(fixed-point type=w1698, number=w1700) -> (fixed-point=w1699:fxp<+/-,58,25>)
                    }
                    frame "Data Log 2" {
                      n435 = To Fixed-Point(fixed-point type=w1711, number=w1716) -> (fixed-point=w1718:fxp<+/-,58,25>)
                      n436 = To Fixed-Point(fixed-point type=w1711, number=w1717) -> (fixed-point=w1710:fxp<+/-,58,25>)
                      n437 = To Fixed-Point(fixed-point type=w1711, number=w1713) -> (fixed-point=w1719:fxp<+/-,58,25>)
                      n438 = To Fixed-Point(fixed-point type=w1711, number=w1712) -> (fixed-point=w1715:fxp<+/-,58,25>)
                      n439 = To Fixed-Point(fixed-point type=w1711, number=w1712) -> (fixed-point=w1709:fxp<+/-,58,25>)
                    }
                    frame "Data Log 3" {
                      n440 = To Fixed-Point(fixed-point type=w1720, number=w1726) -> (fixed-point=w1730:fxp<+/-,58,25>)
                      n441 = To Fixed-Point(fixed-point type=w1720, number=w1727) -> (fixed-point=w1729:fxp<+/-,58,25>)
                      n442 = To Fixed-Point(fixed-point type=w1720, number=w1723) -> (fixed-point=w1728:fxp<+/-,58,25>)
                      n443 = To Fixed-Point(fixed-point type=w1720, number=w1722) -> (fixed-point=w1725:fxp<+/-,58,25>)
                      n444 = To Fixed-Point(fixed-point type=w1720, number=w1722) -> (fixed-point=w1721:fxp<+/-,58,25>)
                    }
                    frame "Data Log 4" {
                      n445 = To Fixed-Point(fixed-point type=w1733, number=w1737) -> (fixed-point=w1741:fxp<+/-,58,25>)
                      n446 = To Fixed-Point(fixed-point type=w1733, number=w1736) -> (fixed-point=w1735:fxp<+/-,58,25>)
                      n447 = To Fixed-Point(fixed-point type=w1733, number=w1734) -> (fixed-point=w1740:fxp<+/-,58,25>)
                      n448 = To Fixed-Point(fixed-point type=w1733, number=w1731) -> (fixed-point=w1739:fxp<+/-,58,25>)
                      n449 = To Fixed-Point(fixed-point type=w1733, number=w1731) -> (fixed-point=w1732:fxp<+/-,58,25>)
                    }
                    frame "Data Log 5" {
                      n450 = To Fixed-Point(fixed-point type=w1742, number=w1747) -> (fixed-point=w1754:fxp<+/-,58,25>)
                      n451 = Subtract(x=w1749, y=w1748) -> (x-y=w1745:fxp<+/-,59,26>)
                      n452 = To Fixed-Point(fixed-point type=w1742, number=w1746) -> (fixed-point=w1753:fxp<+/-,58,25>)
                      n453 = To Fixed-Point(fixed-point type=w1742, number=w1745) -> (fixed-point=w1752:fxp<+/-,58,25>)
                      n454 = To Fixed-Point(fixed-point type=w1742, number=w1744) -> (fixed-point=w1751:fxp<+/-,58,25>)
                      n455 = To Fixed-Point(fixed-point type=w1742, number=w1744) -> (fixed-point=w1743:fxp<+/-,58,25>)
                    }
                    frame "Data Log 6" {
                      n456 = To Fixed-Point(fixed-point type=w1757, number=w1762) -> (fixed-point=w1767:fxp<+/-,58,25>)
                      n457 = To Fixed-Point(fixed-point type=w1757, number=w1761) -> (fixed-point=w1766:fxp<+/-,58,25>)
                      n458 = Subtract(x=w1760, y=w1759) -> (x-y=w1758:fxp<+/-,59,26>)
                      n459 = To Fixed-Point(fixed-point type=w1757, number=w1758) -> (fixed-point=w1765:fxp<+/-,58,25>)
                      n460 = To Fixed-Point(fixed-point type=w1757, number=w1756) -> (fixed-point=w1764:fxp<+/-,58,25>)
                      n461 = To Fixed-Point(fixed-point type=w1757, number=w1756) -> (fixed-point=w1755:fxp<+/-,58,25>)
                    }
                    frame "Data Log 7" {
                      n462 = To Fixed-Point(fixed-point type=w1770, number=w1778) -> (fixed-point=w1777:fxp<+/-,58,25>)
                      n463 = To Fixed-Point(fixed-point type=w1770, number=w1774) -> (fixed-point=w1776:fxp<+/-,58,25>)
                      n464 = Subtract(x=w1773, y=w1772) -> (x-y=w1780:fxp<+/-,59,26>)
                      n465 = To Fixed-Point(fixed-point type=w1770, number=w1780) -> (fixed-point=w1775:fxp<+/-,58,25>)
                      n466 = To Fixed-Point(fixed-point type=w1770, number=w1768) -> (fixed-point=w1771:fxp<+/-,58,25>)
                      n467 = To Fixed-Point(fixed-point type=w1770, number=w1768) -> (fixed-point=w1769:fxp<+/-,58,25>)
                    }
                    frame "Data Log 8" {
                      n468 = Subtract(x=w1797, y=w1796) -> (x-y=w1795:fxp<+/-,59,26>)
                      n469 = Subtract(x=w1793, y=w1792) -> (x-y=w1791:fxp<+/-,59,26>)
                      n470 = To Fixed-Point(fixed-point type=w1782, number=w1795) -> (fixed-point=w1794:fxp<+/-,58,25>)
                      n471 = Subtract(x=w1789, y=w1788) -> (x-y=w1787:fxp<+/-,59,26>)
                      n472 = To Fixed-Point(fixed-point type=w1782, number=w1791) -> (fixed-point=w1790:fxp<+/-,58,25>)
                      n473 = To Fixed-Point(fixed-point type=w1782, number=w1787) -> (fixed-point=w1786:fxp<+/-,58,25>)
                      n474 = To Fixed-Point(fixed-point type=w1782, number=w1781) -> (fixed-point=w1785:fxp<+/-,58,25>)
                      n475 = To Fixed-Point(fixed-point type=w1782, number=w1781) -> (fixed-point=w1783:fxp<+/-,58,25>)
                    }
                    frame "Data Log 9" {
                      n476 = To Fixed-Point(fixed-point type=w1800, number=w1807) -> (fixed-point=w1804:fxp<+/-,58,25>)
                      n477 = To Fixed-Point(fixed-point type=w1800, number=w1806) -> (fixed-point=w1803:fxp<+/-,58,25>)
                      n478 = To Fixed-Point(fixed-point type=w1800, number=w1805) -> (fixed-point=w1802:fxp<+/-,58,25>)
                      n479 = To Fixed-Point(fixed-point type=w1800, number=w1798) -> (fixed-point=w1801:fxp<+/-,58,25>)
                      n480 = To Fixed-Point(fixed-point type=w1800, number=w1798) -> (fixed-point=w1799:fxp<+/-,58,25>)
                    }
                    frame "Data Log 10" {
                      n481 = To Fixed-Point(fixed-point type=w1812, number=w1819) -> (fixed-point=w1818:fxp<+/-,58,25>)
                      n482 = To Fixed-Point(fixed-point type=w1812, number=w1817) -> (fixed-point=w1813:fxp<+/-,58,25>)
                      n483 = To Fixed-Point(fixed-point type=w1812, number=w1816) -> (fixed-point=w1814:fxp<+/-,58,25>)
                      n484 = To Fixed-Point(fixed-point type=w1812, number=w1810) -> (fixed-point=w1815:fxp<+/-,58,25>)
                      n485 = To Fixed-Point(fixed-point type=w1812, number=w1809) -> (fixed-point=w1811:fxp<+/-,58,25>)
                    }
                    frame "Data Log 11" {
                      n486 = To Fixed-Point(fixed-point type=w1822, number=w1832) -> (fixed-point=w1827:fxp<+/-,58,25>)
                      n487 = To Fixed-Point(fixed-point type=w1822, number=w1831) -> (fixed-point=w1826:fxp<+/-,58,25>)
                      n488 = To Fixed-Point(fixed-point type=w1822, number=w1830) -> (fixed-point=w1825:fxp<+/-,58,25>)
                      n489 = To Fixed-Point(fixed-point type=w1822, number=w1829) -> (fixed-point=w1824:fxp<+/-,58,25>)
                      n490 = To Fixed-Point(fixed-point type=w1822, number=w1821) -> (fixed-point=w1823:fxp<+/-,58,25>)
                    }
                    frame "Data Log 12" {
                      n491 = To Fixed-Point(fixed-point type=w1834, number=w1843) -> (fixed-point=w1842:fxp<+/-,58,25>)
                      n492 = To Fixed-Point(fixed-point type=w1834, number=w1838) -> (fixed-point=w1841:fxp<+/-,58,25>)
                      n493 = To Fixed-Point(fixed-point type=w1834, number=w1837) -> (fixed-point=w1840:fxp<+/-,58,25>)
                      n494 = To Fixed-Point(fixed-point type=w1834, number=w1836) -> (fixed-point=w1839:fxp<+/-,58,25>)
                      n495 = To Fixed-Point(fixed-point type=w1834, number=w1833) -> (fixed-point=w1835:fxp<+/-,58,25>)
                    }
                    frame "Data Log 13" {
                      n496 = To Fixed-Point(fixed-point type=w1845, number=w1850) -> (fixed-point=w1854:fxp<+/-,58,25>)
                      n497 = To Fixed-Point(fixed-point type=w1845, number=w1849) -> (fixed-point=w1853:fxp<+/-,58,25>)
                      n498 = To Fixed-Point(fixed-point type=w1845, number=w1848) -> (fixed-point=w1852:fxp<+/-,58,25>)
                      n499 = To Fixed-Point(fixed-point type=w1845, number=w1847) -> (fixed-point=w1851:fxp<+/-,58,25>)
                      n500 = To Fixed-Point(fixed-point type=w1845, number=w1847) -> (fixed-point=w1846:fxp<+/-,58,25>)
                    }
                    frame "Data Log 14" {
                      n501 = To Fixed-Point(fixed-point type=w1857, number=w1861) -> (fixed-point=w1865:fxp<+/-,58,25>)
                      n502 = To Fixed-Point(fixed-point type=w1857, number=w1860) -> (fixed-point=w1864:fxp<+/-,58,25>)
                      n503 = To Fixed-Point(fixed-point type=w1857, number=w1859) -> (fixed-point=w1863:fxp<+/-,58,25>)
                      n504 = To Fixed-Point(fixed-point type=w1857, number=w1856) -> (fixed-point=w1862:fxp<+/-,58,25>)
                      n505 = To Fixed-Point(fixed-point type=w1857, number=w1856) -> (fixed-point=w1858:fxp<+/-,58,25>)
                    }
                    frame "Data Log 15" {
                      n506 = To Fixed-Point(fixed-point type=w1868, number=w1872) -> (fixed-point=w1876:fxp<+/-,58,25>)
                      n507 = To Fixed-Point(fixed-point type=w1868, number=w1871) -> (fixed-point=w1875:fxp<+/-,58,25>)
                      n508 = To Fixed-Point(fixed-point type=w1868, number=w1870) -> (fixed-point=w1874:fxp<+/-,58,25>)
                      n509 = To Fixed-Point(fixed-point type=w1868, number=w1867) -> (fixed-point=w1873:fxp<+/-,58,25>)
                      n510 = To Fixed-Point(fixed-point type=w1868, number=w1867) -> (fixed-point=w1869:fxp<+/-,58,25>)
                    }
                    frame "Data Log 16" {
                      n511 = To Fixed-Point(fixed-point type=w1880, number=w1884) -> (fixed-point=w1888:fxp<+/-,58,25>)
                      n512 = To Fixed-Point(fixed-point type=w1880, number=w1883) -> (fixed-point=w1887:fxp<+/-,58,25>)
                      n513 = To Fixed-Point(fixed-point type=w1880, number=w1882) -> (fixed-point=w1886:fxp<+/-,58,25>)
                      n514 = To Fixed-Point(fixed-point type=w1880, number=w1881) -> (fixed-point=w1885:fxp<+/-,58,25>)
                      n515 = To Fixed-Point(fixed-point type=w1880, number=w1879) -> (fixed-point=w1878:fxp<+/-,58,25>)
                    }
                  }
                  "Number of Data Strings" <- w1677
                  n516 = Build Array "Build Array"(w1691, w1690, w1689, w1679, w1671) -> (w1673:fxp<+/-,58,25>[])
                }
              }
            }
          }
          n517 = call "Loop Timer2"("Count(uSec)"="Datalog Time Period (uSec)") -> ()  [unwired: 1 out]
          n518 = for {
            N: w1654 -> [_]
            tunnel: w1647 -> [w1897] mode=indexing
            shift-right: [w1895] -> w1653
            shift-left: _ -> [w1894]
            shift-right: [w1891] -> w1648
            shift-left: _ -> [w1892]
            n519 = xnode "FIFO"("Element"=w1897, "Timeout"="Timeout FPGA FIFO1", "error in (no error)"=w1894) -> ("Timed Out?"=w1893:bool, "error out"=w1895:errorcluster)  [unwired: 1 in, 1 out]
            "FIFO Timed Out?" <- w1893
            n520 = Or(x=w1893, y=w1892) -> (x .or. y?=w1891:bool)
          }
          "FIFO Timed Out" <- w1648
          n521 = call "measure_loop_rate_FPGA.vi"() -> ("Loop Rate (Ticks)"=→"Measured Datalog Time Period (Ticks)":u32)  [unwired: 11 in]
          n522 = local read "stop case"() -> (w1649:bool)
          n523 = local read "Y scan done"() -> (w1639:bool)
          n524 = local read "X scan done"() -> (w1638:bool)
          n525 = Unbundle By Name "Unbundle By Name"(w1653) -> ("Status?"=w1652:bool)
          n526 = And(x=w1639, y=w1638) -> (x .and. y?=w1637:bool)
          "Fly scan completed" <- w1637
          n527 = Compound Arithmetic op=OR(w1652, w1648, w1649, w1637) -> (w1651:bool)
          n528 = case shown="True" w1651 {
            selector: w1651 -> [_ w1890]
            frame False {
            }
            frame True {
              n529 = local write "stop case"(w1890) -> ()
            }
          }
        }
        n530 = while {
          stop <- w578 stop-if-true
          w557 = fxp<+/-,58,25> 0.0 ("fixed-point type")
          n531 = local read "32 bit Count Sample  Y"() -> (w554:i32)
          n532 = local read "32 bit Count Sample  Z"() -> (w551:i32)
          n533 = local read "32 bit Count Sample X"() -> (w555:i32)
          n534 = local read "32 bit Count Optics  Y"() -> (w571:i32)
          n535 = local read "32 bit Count Optics  Z"() -> (w567:i32)
          n536 = local read "32 bit Count Optics X"() -> (w577:i32)
          n537 = Multiply(x=w577, y="Optics X Stage Resolution (nm)") -> (x*y=w574:fxp<+/-,64,35>)
          "Optics X Stage Displacement raw (nm)" <- w574
          n538 = Multiply(x=w555, y="Sample X Stage Resolution (nm)") -> (x*y=w563:fxp<+/-,64,35>)
          "Sample X Stage Displacement raw (nm)" <- w563
          n539 = Multiply(x=w571, y="Optics Y Stage Resolution (nm)") -> (x*y=w569:fxp<+/-,64,35>)
          "Optics Y Stage Displacement raw (nm)" <- w569
          n540 = Multiply(x=w554, y="Sample Y Stage Resolution (nm)") -> (x*y=w561:fxp<+/-,64,35>)
          "Sample Y Stage Displacement raw (nm)" <- w561
          n541 = Multiply(x=w567, y="Optics Z Stage Resolution (nm)") -> (x*y=w565:fxp<+/-,64,35>)
          "Optics Z Stage Displacement raw (nm)" <- w565
          n542 = Multiply(x=w551, y="Sample Z Stage Resolution (nm)") -> (x*y=w559:fxp<+/-,64,35>)
          "Sample Z Stage Displacement raw (nm)" <- w559
          n543 = call "Loop Timer5"("Count(uSec)"="Plant Output Time Period (uSec)") -> ()  [unwired: 1 out]
          n544 = call "measure_loop_rate_FPGA.vi"() -> ("Loop Rate (Ticks)"=→"Measured Plant Output Time Period (Ticks)":u32)  [unwired: 11 in]
          n545 = To Fixed-Point(fixed-point type=w557, number=w574) -> (fixed-point=→"Optics X Stage Displacement (nm)":fxp<+/-,58,25>)
          n546 = To Fixed-Point(fixed-point type=w557, number=w569) -> (fixed-point=→"Optics Y Stage Displacement (nm)":fxp<+/-,58,25>)
          n547 = To Fixed-Point(fixed-point type=w557, number=w565) -> (fixed-point=→"Optics Z Stage Displacement (nm)":fxp<+/-,58,25>)
          n548 = To Fixed-Point(fixed-point type=w557, number=w563) -> (fixed-point=→"Sample X Stage Displacement (nm)":fxp<+/-,58,25>)
          n549 = To Fixed-Point(fixed-point type=w557, number=w561) -> (fixed-point=→"Sample Y Stage Displacement (nm)":fxp<+/-,58,25>)
          n550 = To Fixed-Point(fixed-point type=w557, number=w559) -> (fixed-point=→"Sample Z Stage Displacement (nm)":fxp<+/-,58,25>)
          n551 = local read "stop case"() -> (w578:bool)
        }
        n552 = timed-loop {
          timing: w119 -> [_]
          timing-out: [_] -> w118
          tunnel: [w579] -> w112
          shift-right: [w676] -> _
          shift-left: _ -> [w585]
          shift-right: [w675] -> _
          shift-left: _ -> [w674]
          shift-right: [w673] -> w92
          shift-left: w98 -> [w672]
          shift-right: [w671] -> _
          shift-left: u32 0 ("Tick Count(Ticks)") -> [w670]
          tunnel: [w669] -> w117
          shift-right: [w657] -> _
          shift-left: _ -> [w655]
          shift-right: [w656] -> _
          shift-left: _ -> [w654]
          shift-right: [w653] -> w90
          shift-left: w96 -> [w652]
          shift-right: [w640] -> _
          shift-left: _ -> [w638]
          shift-right: [w639] -> _
          shift-left: _ -> [w637]
          shift-right: [w636] -> w88
          shift-left: w94 -> [w635]
          shift-right: [w623] -> _
          shift-left: _ -> [w620]
          shift-right: [w622] -> _
          shift-left: _ -> [w621]
          shift-right: [w619] -> w91
          shift-left: w97 -> [w618]
          shift-right: [w606] -> _
          shift-left: _ -> [w603]
          shift-right: [w605] -> _
          shift-left: _ -> [w604]
          shift-right: [w602] -> w89
          shift-left: w95 -> [w601]
          tunnel: [w588] -> _
          shift-right: [w589] -> _
          shift-left: _ -> [w587]
          shift-right: [w588] -> _
          shift-left: _ -> [w586]
          shift-right: [w584] -> w87
          shift-left: w93 -> [w583]
          stop <- w581 stop-if-true
          n553 = xnode "FPGA I/O Node"() -> ("error out"=w579:errorcluster, "Mod4/DIO0"=w676:bool, "Mod4/DIO1"=w675:bool, "Mod4/DIO2"=w623:bool, "Mod4/DIO3"=w622:bool, "Mod5/DIO0"=w657:bool, "Mod5/DIO1"=w656:bool, "Mod5/DIO2"=w606:bool, "Mod5/DIO3"=w605:bool, "Mod6/DIO0"=w640:bool, "Mod6/DIO1"=w639:bool, "Mod6/DIO2"=w589:bool, "Mod6/DIO3"=w588:bool)  [unwired: 13 in, 12 out]
          "Mod4/DIO0" <- w676
          "Mod4/DIO1" <- w675
          "Mod5/DIO0" <- w657
          "Mod5/DIO1" <- w656
          "Mod6/DIO0" <- w640
          "Mod6/DIO1" <- w639
          "Mod4/DIO2" <- w623
          "Mod4/DIO3" <- w622
          "Mod5/DIO2" <- w606
          "Mod5/DIO3" <- w605
          "Mod6/DIO2" <- w589
          "Mod6/DIO3" <- w588
          n554 = Exclusive Or(1:w586, 2:w589) -> (0:w590:bool)
          n555 = Exclusive Or(1:w637, 2:w640) -> (0:w641:bool)
          n556 = Exclusive Or(1:w654, 2:w657) -> (0:w658:bool)
          n557 = Exclusive Or(1:w604, 2:w606) -> (0:w607:bool)
          n558 = call "Tick Count"() -> ("Tick Count(Ticks)"=w671:u32)
          n559 = Exclusive Or(1:w674, 2:w676) -> (0:w677:bool)
          n560 = Exclusive Or(1:w621, 2:w623) -> (0:w624:bool)
          n561 = Select(t=0, s="Reset Sample Z", f=w583) -> (s? t:f=w599:i32)
          n562 = Select(t=0, s="Reset Optics Z", f=w635) -> (s? t:f=w650:i32)
          n563 = Select(t=0, s="Reset Optics Y", f=w652) -> (s? t:f=w667:i32)
          n564 = Exclusive Or(1:w586, 2:w588) -> (0:w596:bool)
          n565 = Exclusive Or(1:w637, 2:w639) -> (0:w647:bool)
          n566 = Exclusive Or(1:w654, 2:w656) -> (0:w664:bool)
          n567 = Select(t=0, s="Reset Sample Y", f=w601) -> (s? t:f=w616:i32)
          n568 = Exclusive Or(1:w604, 2:w605) -> (0:w613:bool)
          n569 = Exclusive Or(1:w587, 2:w589) -> (0:w595:bool)
          n570 = Exclusive Or(1:w638, 2:w640) -> (0:w646:bool)
          n571 = Exclusive Or(1:w655, 2:w657) -> (0:w663:bool)
          n572 = Select(t=1 ("x"), s=w590, f=-1 ("x")) -> (s? t:f=w592:i32)
          n573 = Select(t=1 ("x"), s=w641, f=-1 ("x")) -> (s? t:f=w643:i32)
          n574 = Select(t=1 ("x"), s=w658, f=-1 ("x")) -> (s? t:f=w660:i32)
          n575 = Exclusive Or(1:w603, 2:w606) -> (0:w612:bool)
          n576 = Subtract(x=w671, y=w670) -> (x-y=w669:u32)
          n577 = Select(t=0, s="Reset Optics X", f=w672) -> (s? t:f=w686:i32)
          n578 = Select(t=1 ("x"), s=w607, f=-1 ("x")) -> (s? t:f=w609:i32)
          n579 = Select(t=0, s="Reset Sample X", f=w618) -> (s? t:f=w633:i32)
          n580 = Exclusive Or(1:w674, 2:w675) -> (0:w683:bool)
          n581 = Exclusive Or(1:w621, 2:w622) -> (0:w630:bool)
          n582 = Or(x=w595, y=w596) -> (x .or. y?=w594:bool)
          n583 = Or(x=w646, y=w647) -> (x .or. y?=w645:bool)
          n584 = Or(x=w663, y=w664) -> (x .or. y?=w662:bool)
          n585 = Exclusive Or(1:w585, 2:w676) -> (0:w682:bool)
          n586 = Exclusive Or(1:w620, 2:w623) -> (0:w629:bool)
          n587 = Or(x=w612, y=w613) -> (x .or. y?=w611:bool)
          n588 = Select(t=1 ("x"), s=w677, f=-1 ("x")) -> (s? t:f=w679:i32)
          n589 = Select(t=1 ("x"), s=w624, f=-1 ("x")) -> (s? t:f=w626:i32)
          n590 = Or(x=w682, y=w683) -> (x .or. y?=w681:bool)
          n591 = Or(x=w629, y=w630) -> (x .or. y?=w628:bool)
          n592 = Add(x=w592, y=w599) -> (x+y=w600:i32)
          n593 = Add(x=w643, y=w650) -> (x+y=w651:i32)
          n594 = Add(x=w660, y=w667) -> (x+y=w668:i32)
          n595 = Add(x=w609, y=w616) -> (x+y=w617:i32)
          n596 = Select(t=w600, s=w594, f=w599) -> (s? t:f=w584:i32)
          "32 bit Count Sample  Z" <- w584
          n597 = Select(t=w651, s=w645, f=w650) -> (s? t:f=w636:i32)
          "32 bit Count Optics  Z" <- w636
          n598 = Select(t=w668, s=w662, f=w667) -> (s? t:f=w653:i32)
          "32 bit Count Optics  Y" <- w653
          n599 = Add(x=w679, y=w686) -> (x+y=w687:i32)
          n600 = Add(x=w626, y=w633) -> (x+y=w634:i32)
          n601 = Select(t=w617, s=w611, f=w616) -> (s? t:f=w602:i32)
          "32 bit Count Sample  Y" <- w602
          n602 = Select(t=w687, s=w681, f=w686) -> (s? t:f=w673:i32)
          "32 bit Count Optics X" <- w673
          n603 = local read "stop case"() -> (w580:bool)
          n604 = Select(t=w634, s=w628, f=w633) -> (s? t:f=w619:i32)
          "32 bit Count Sample X" <- w619
          n605 = Unbundle By Name(w579) -> ("status"=w582:bool)
          n606 = Or(x=w582, y=w580) -> (x .or. y?=w581:bool)
        }
        "Measured Counter Time Period (Ticks)" <- w117
        n607 = while {
          tunnel: [w531] -> w109
          stop <- w529 stop-if-true
          w536 = fxp<+/-,58,25> 0.0 ("fixed-point type")
          n608 = xnode "FPGA I/O Node"("FPGA I/O In"=refnum<k21> "Mod3/AI0", "FPGA I/O In"=refnum<k21> "Mod3/AI1", "FPGA I/O In"=refnum<k21> "Mod3/AI2") -> ("error out"=w531:errorcluster, "I/O Item"=w547:fxp<+/-,24,5>, "I/O Item"=w538:fxp<+/-,24,5>, "I/O Item"=w537:fxp<+/-,24,5>)  [unwired: 1 in, 3 out]
          "Mod 3 Input AI0 (V)" <- w547
          "Mod 8 Input AI1 (V)" <- w538
          "Mod 8 Input AI2 (V)" <- w537
          n609 = call "Loop Timer6"("Count(uSec)"="Analog Input Time Period (uSec)") -> ()  [unwired: 1 out]
          n610 = Multiply(x=w537, y="Mod 3 AI2 V to nm Scaling") -> (x*y=w540:fxp<+/-,64,23>)
          n611 = Multiply(x=w538, y="Mod 3 AI1 V to nm Scaling") -> (x*y=w543:fxp<+/-,64,23>)
          n612 = Multiply(x=w547, y="Mod 3 AI0 V to nm Scaling") -> (x*y=w549:fxp<+/-,64,23>)
          n613 = To Fixed-Point(fixed-point type=w536, number=w549) -> (fixed-point=→"X Stage External Reference (nm)":fxp<+/-,58,25>)
          n614 = To Fixed-Point(fixed-point type=w536, number=w543) -> (fixed-point=→"Y Stage External Reference (nm)":fxp<+/-,58,25>)
          n615 = To Fixed-Point(fixed-point type=w536, number=w540) -> (fixed-point=→"Z Stage External Reference (nm)":fxp<+/-,58,25>)
          n616 = call "measure_loop_rate_FPGA.vi"() -> ("Loop Rate (Ticks)"=→"Measured Analog Input Time Period (Ticks)":u32)  [unwired: 11 in]
          n617 = local read "stop case"() -> (w530:bool)
          n618 = Unbundle By Name(w531) -> ("status"=w532:bool)
          n619 = Or(x=w532, y=w530) -> (x .or. y?=w529:bool)
        }
        n620 = while {
          tunnel: [w697] -> w110
          stop <- w699 stop-if-true
          n621 = local read "PI X-Stage Input (V)"() -> (w706:fxp<+/-,20,5>)
          n622 = local read "PI Y-Stage Input (V)"() -> (w705:fxp<+/-,20,5>)
          n623 = local read "PI Z-Stage Input (V)"() -> (w704:fxp<+/-,20,5>)
          n624 = xnode "FPGA I/O Node"("I/O Item"=w706, "FPGA I/O In"=refnum<k21> "Mod8/AO0", "I/O Item"=w705, "FPGA I/O In"=refnum<k21> "Mod8/AO1") -> ("error out"=w703:errorcluster)  [unwired: 1 in, 2 out]
          n625 = xnode "FPGA I/O Node"("I/O Item"=w704, "FPGA I/O In"=refnum<k21> "Mod8/AO2") -> ("error out"=w707:errorcluster)  [unwired: 1 in, 1 out]
          n626 = call "Loop Timer4"("Count(uSec)"="Controller Output Time Period (uSec)") -> ()  [unwired: 1 out]
          n627 = Merge Errors "Merge Errors"(w703, w707) -> (w697:errorcluster)
          n628 = call "measure_loop_rate_FPGA.vi"() -> ("Loop Rate (Ticks)"=→"Measured Controller Output Time Period (Ticks)":u32)  [unwired: 11 in]
          n629 = local read "stop case"() -> (w698:bool)
          n630 = Unbundle By Name(w697) -> ("status"=w696:bool)
          n631 = Or(x=w696, y=w698) -> (x .or. y?=w699:bool)
        }
        n632 = while {
          stop <- w123 stop-if-true
          n633 = local read "DT Frequency (periods/tick)"() -> (w127:fxp<+,32,0>)
          n634 = local read "DT Phase Offset (periods)"() -> (w126:fxp<+,32,0>)
          n635 = local read "DT Duty Cycle (periods)"() -> (w125:fxp<+,32,0>)
          n636 = local read "DT Reset"() -> (w124:bool)
          n637 = call "Square Wave Generator2"("frequency (periods/tick)"=w127, "reset"=w124, "phase offset (periods)"=w126, "duty cycle (periods)"=w125) -> ("square wave out"=w134:i16)  [unwired: 11 in]
          n638 = call "Loop Timer11"("Count(uSec)"="Data Trigger Time Period (uSec)") -> ()  [unwired: 1 out]
          n639 = call "measure_loop_rate_FPGA.vi"() -> ("Loop Rate (Ticks)"=→"Measured Data Trigger Time Period (Ticks)":u32)  [unwired: 11 in]
          n640 = Divide(x=w134, y=i16 32767) -> (x/y=w130:fxp<+/-,41,18>)
          n641 = To Fixed-Point(fixed-point type=fxp<+/-,58,25> 0.0, number=w130) -> (fixed-point=→"Trigger for Data":fxp<+/-,58,25>)
          n642 = local read "stop case"() -> (w123:bool)
        }
        n643 = node-c288(w118) -> (w113:errorcluster)
        n644 = while {
          tunnel: [w380] -> w108
          stop <- w385 stop-if-true
          n645 = local read "Detector Trigger (V)"() -> (w381:fxp<+/-,20,5>)
          n646 = call "Loop Timer8"("Count(uSec)"="Detector Trigger Time Period (uSec)") -> ()  [unwired: 1 out]
          n647 = call "measure_loop_rate_FPGA.vi"() -> ("Loop Rate (Ticks)"=→"Measured Detector Trigger Time Period (Ticks)":u32)  [unwired: 11 in]
          n648 = xnode "FPGA I/O Node"("I/O Item"=w381, "FPGA I/O In"=refnum<k21> "Mod8/AO3") -> ("error out"=w380:errorcluster)  [unwired: 1 in, 1 out]
          n649 = local read "stop case"() -> (w385:bool)
        }
        n650 = Merge Errors(w108, w110, w109, w113, w112, w114) -> (w99:errorcluster)
        "Run Loop error" <- w99
        n651 = case shown="No Error" w99 {
          tunnel: [FPGA_states."End Run" FPGA_states."Wait"] -> w100
          frame No Error {
          }
          frame Error {
            n652 = local write "stop case"(TRUE) -> ()
          }
        }
      }
      frame "End Run" {
        n653 = xnode "FPGA I/O Node"("Mod3/Stop"=TRUE ("I/O Item")) -> ("error out"=w2049:errorcluster)  [unwired: 2 in, 1 out]
        "End Run Error" <- w2049
      }
      frame "Shutdown" {
        n654 = xnode "FPGA I/O Node"("error in"=w2060, "System Reset"=TRUE) -> ("error out"=w2059:errorcluster)  [unwired: 1 in, 1 out]
        "Shutdown error" <- w2059
      }
    }
    "FPGA state" <- w45
  }
